vi "J1939 System Definition API_Example_Create Sysdef and Add J1939 CD.vi"(8 "error in (no error)":errorcluster) -> (0 "error out":errorcluster, 3 "Sysdef Path":path=path "C:/Users/Public/Documents/National Instruments/NI VeriStand 2011/Projects/DynamicallyCreatedProject/DynamicallyCreatedProject.nivssdf")   [LabVIEW 2013]
uses:
  J1939 System Definition API.lvlibp/APIs/System Definition API/Types/Add Item - Frame Cluster.ctl
  J1939 System Definition API.lvlibp/APIs/System Definition API/Types/Remove Frame Action.ctl
  J1939 System Definition API.lvlibp/Shared/Types/XNET Settings.ctl
  J1939 System Definition API.lvlibp/Shared/Types/Monitor Settings.ctl
  NationalInstruments.VeriStand.SystemDefinitionAPI
  J1939 System Definition API.lvlibp/APIs/System Definition API/SubVIs/Add Frames.vi
  J1939 System Definition API.lvlibp/APIs/System Definition API/SubVIs/Add Device.vi
  J1939 System Definition API.lvlibp/APIs/System Definition API/SubVIs/Add DTC.vi
  J1939 System Definition API.lvlibp
  J1939 System Definition API.lvlibp/APIs/System Definition API/J1939 System Definition API Support.lvlib
  J1939 System Definition API.lvlibp/Shared/J1939 Addon Shared.lvlib
panel:
  in  "Outgoing Frames":T1[](array[typedef])=[{"XNET Frame"="A1\nj1939", "Signals"=["EngBlowerBypassValvePos\nj1939", "EngGasSupplyPress\nj1939"]}, {"XNET Frame"="AAC1\nj1939", "Signals"=["Aftertreatment1AirPressCtrl\nj1939", "Aftertreatment1AirSystemRelay\nj1939", "Aftertreatment1PurgeAirActuator\nj1939", "Aftertreatment1PurgeAirPress\nj1939", "Aftertreatment1SupplyAirPress\nj1939", "Aftrtreatment1AirEnableActuator\nj1939", "Aftrtrtment1AirPressActuatorPos\nj1939", "Aftrtrtmnt1AtmzationAirActuator\nj1939"]}, {"XNET Frame"="AAC2\nj1939", "Signals"=["Aftertreatment2AirPressCtrl\nj1939", "Aftertreatment2AirSystemRelay\nj1939", "Aftertreatment2PurgeAirActuator\nj1939", "Aftertreatment2PurgeAirPress\nj1939", "Aftertreatment2SupplyAirPress\nj1939", "Aftrtreatment2AirEnableActuator\nj1939", "Aftrtrtment2AirPressActuatorPos\nj1939", "Aftrtrtmnt2AtmzationAirActuator\nj1939"]}, {"XNET Frame"="AAC3\nj1939", "Signals"=["Aftertreatment1SecondAirPress\nj1939", "Aftertreatment1SecondAirTemp\nj1939", "Aftrtratment1SecondAirDiffPress\nj1939", "Aftrtreatment1SecondAirMassFlow\nj1939"]}, {"XNET Frame"="AAC4\nj1939", "Signals"=["Aftertreatment2SecondAirPress\nj1939", "Aftertreatment2SecondAirTemp\nj1939", "Aftrtratment2SecondAirDiffPress\nj1939", "Aftrtreatment2SecondAirMassFlow\nj1939"]}, {"XNET Frame"="AAI\nj1939", "Signals"=["AuxLevel\nj1939", "AuxPress1\nj1939", "AuxPress2\nj1939", "AuxTemp1\nj1939", "AuxTemp2\nj1939"]}, {"XNET Frame"="AC\nj1939", "Signals"=["ArticulationAngle\nj1939"]}, {"XNET Frame"="ACC1\nj1939", "Signals"=["ACCDistanceAlertSignal\nj1939", "ACCSystemShutoffWarning\nj1939", "ACCTargetDetected\nj1939", "AdaptiveCruiseCtrlMode\nj1939", "AdaptiveCruiseCtrlSetSpeed\nj1939", "AdptveCruiseCtrlSetDistanceMode\nj1939", "DistanceToForwardVehicle\nj1939", "ACC1.RoadCurvature\nj1939", "SpeedOfForwardVehicle\nj1939"]}, {"XNET Frame"="ACC2\nj1939", "Signals"=["RqedACCDistanceMode\nj1939"]}, {"XNET Frame"="ACKM\nj1939", "Signals"=["AddressAccessDenied\nj1939", "AddressAcknowledged\nj1939", "AddressBusy\nj1939", "AddressNegativeAcknowledgement\nj1939", "ACKM.ControlByte\nj1939", "GroupFunctionValue\nj1939", "ACKM.ParameterGroupNumber\nj1939"]}, {"XNET Frame"="ACL\nj1939", "Signals"=["ACL.ArbitraryAddressCapable\nj1939", "ACL.ECUInstance\nj1939", "ACL.Function\nj1939", "ACL.FunctionInstance\nj1939", "ACL.IdentityNumber\nj1939", "ACL.IndustryGroup\nj1939", "ACL.ManufacturerCode\nj1939", "ACL.VehicleSystem\nj1939", "ACL.VehicleSystemInstance\nj1939"]}, {"XNET Frame"="AETC\nj1939", "Signals"=["AETCDataCollectionStandard\nj1939", "NumberOfAETCDataPoints\nj1939"]}, {"XNET Frame"="AF2\nj1939", "Signals"=["EngDsiredAbsIntakeManifoldPress\nj1939", "EngGasFuelCorrectionFactor\nj1939", "EngGsMssFlwSnsrFelingCorrection\nj1939", "EngTurboWastegateValvePos\nj1939"]}, {"XNET Frame"="AFC1\nj1939", "Signals"=["Aftertreatment1FuelPress\nj1939", "Aftertreatment1FuelPressCtrl\nj1939", "Aftertreatment1FuelRate\nj1939", "Aftertreatment1Ignt\nj1939", "Aftrtratment1FuelEnableActuator\nj1939", "Aftrtratment1RegenerationStatus\nj1939"]}, {"XNET Frame"="AFC2\nj1939", "Signals"=["Aftertreatment2FuelPress\nj1939", "Aftertreatment2FuelPressCtrl\nj1939", "Aftertreatment2FuelRate\nj1939", "Aftertreatment2Ignt\nj1939", "Aftrtratment2FuelEnableActuator\nj1939", "Aftrtratment2RegenerationStatus\nj1939"]}, {"XNET Frame"="AFSS\nj1939", "Signals"=["LeftHeadlampDynamicBendingLight\nj1939", "LeftHeadlampLightDistribution\nj1939", "RghtHeadlampDynamicBendingLight\nj1939", "RightHeadlampLightDistribution\nj1939"]}, {"XNET Frame"="AI\nj1939", "Signals"=["DriveAxleLiftAirPress\nj1939", "DriveAxleLocation\nj1939", "DriveAxleLubePress\nj1939", "DriveAxleTemp\nj1939", "SteerAxleLubePress\nj1939", "SteerAxleTemp\nj1939"]}, {"XNET Frame"="AIR1\nj1939", "Signals"=["AirCompressorStatus\nj1939", "AirSuspensionSupplyPress\nj1939", "AuxEquipmentSupplyPress\nj1939", "ParkingAnd_OrTrailerAirPress\nj1939", "PneumaticSupplyPress\nj1939", "ServiceBrakeAirPressCircuit1\nj1939", "ServiceBrakeAirPressCircuit2\nj1939"]}, {"XNET Frame"="AIR2\nj1939", "Signals"=["EngAirStartPress\nj1939"]}, {"XNET Frame"="AMB\nj1939", "Signals"=["AmbientAirTemp\nj1939", "BarometricPress\nj1939", "CabInteriorTemp\nj1939", "EngAirInletTemp\nj1939", "RoadSurfaceTemp\nj1939"]}, {"XNET Frame"="AMB2\nj1939", "Signals"=["SolarIntensityPercent\nj1939", "SolarSensorMax\nj1939"]}, {"XNET Frame"="AP\nj1939", "Signals"=["AuxAbsPressReading\nj1939", "AuxGagePressReading1\nj1939", "AuxVacuumPressReading\nj1939"]}, {"XNET Frame"="AS\nj1939", "Signals"=["Alt1Status\nj1939", "Alt2Status\nj1939", "Alt3Status\nj1939", "Alt4Status\nj1939", "AltSpeed\nj1939"]}, {"XNET Frame"="ASC1\nj1939", "Signals"=["AboveNominalLevelFrontAxle\nj1939", "AboveNominalLevelRearAxle\nj1939", "BelowNominalLevelFrontAxle\nj1939", "BelowNominalLevelRearAxle\nj1939", "DoorRelease\nj1939", "FrontAxleInBumperRange\nj1939", "KneelingInformation\nj1939", "LevelCtrlMode\nj1939", "ASC1.LiftAxle1Pos\nj1939", "ASC1.LiftAxle2Pos\nj1939", "LiftingCtrlModeFrontAxle\nj1939", "LiftingCtrlModeRearAxle\nj1939", "LoweringCtrlModeFrontAxle\nj1939", "LoweringCtrlModeRearAxle\nj1939", "NominalLevelFrontAxle\nj1939", "NominalLevelRearAxle\nj1939", "RearAxleInBumperRange\nj1939", "SecurityDevice\nj1939", "SspensionCtrlRefusalInformation\nj1939", "SuspensionRemoteCtrl1\nj1939", "SuspensionRemoteCtrl2\nj1939", "VehicleMotionInhibit\nj1939"]}, {"XNET Frame"="ASC2\nj1939", "Signals"=["AutomaticTractionHelp\nj1939", "DamperStiffnessRqFrontAxle\nj1939", "DamperStiffnessRqLift_TagAxle\nj1939", "DamperStiffnessRqRearAxle\nj1939", "KneelingCmdFrontAxle\nj1939", "KneelingCmdRearAxle\nj1939", "KneelingCtrlModeRq\nj1939", "KneelingRqLeftSide\nj1939", "KneelingRqRightSide\nj1939", "LevelCtrlModeRq\nj1939", "LiftAxle1PosCmd\nj1939", "LiftAxle2PosCmd\nj1939", "NominalLevelRqFrontAxle\nj1939", "NominalLevelRqRearAxle\nj1939", "ProhibitAirSuspensionCtrl\nj1939"]}, {"XNET Frame"="ASC3\nj1939", "Signals"=["RelativeLevelFrontAxleLeft\nj1939", "RelativeLevelFrontAxleRight\nj1939", "RelativeLevelRearAxleLeft\nj1939", "RelativeLevelRearAxleRight\nj1939"]}, {"XNET Frame"="ASC4\nj1939", "Signals"=["BellowPressFrontAxleLeft\nj1939", "BellowPressFrontAxleRight\nj1939", "BellowPressRearAxleLeft\nj1939", "BellowPressRearAxleRight\nj1939"]}, {"XNET Frame"="ASC5\nj1939", "Signals"=["DamperStiffnessFrontAxle\nj1939", "DamperStiffnessLift_TagAxle\nj1939", "DamperStiffnessRearAxle\nj1939", "ElctrncShckAbsrbrCtrlMdFrntAxle\nj1939", "ElctrncShckAbsrbrCtrlMdLft_TgAxl\nj1939", "ElctrncShckAbsrbrCtrlMdRearAxle\nj1939"]}, {"XNET Frame"="ASC6\nj1939", "Signals"=["LevelPresetFrontAxleLeft\nj1939", "LevelPresetFrontAxleRight\nj1939", "LevelPresetRearAxleLeft\nj1939", "LevelPresetRearAxleRight\nj1939"]}, {"XNET Frame"="AT\nj1939", "Signals"=["EngAltBearing1Temp\nj1939", "EngAltBearing2Temp\nj1939", "EngAltWinding1Temp\nj1939", "EngAltWinding2Temp\nj1939", "EngAltWinding3Temp\nj1939"]}, {"XNET Frame"="AT1I1\nj1939", "Signals"=["Aftertreatment1IntakeNOx\nj1939", "Aftertreatment1IntakeO2\nj1939", "Aftrtrtmnt1IntkGsSnsrHeaterCtrl\nj1939", "Aftrtrtmnt1IntkGsSnsrHtrPrlmnryF\nj1939", "Aftrtrtmnt1IntkGsSnsrPwrInRange\nj1939", "Aftrtrtmnt1IntkNOxReadingStable\nj1939", "Aftrtrtmnt1IntkNOxSnsrPrlmnryFMI\nj1939", "Aftrtrtmnt1IntkOxygnSnsrPrlmnryF\nj1939", "Aftrtrtmnt1IntkWdRngO2RdngStble\nj1939", "Aftrtrtmnt1IntkeGasSensorAtTemp\nj1939"]}, {"XNET Frame"="AT1I2\nj1939", "Signals"=["Aftertreatment1ExhaustGasTemp1\nj1939", "Aftrtrtmnt1ExhstGsTmp1PrlmnryFMI\nj1939", "Aftrtrtmnt1PrtcltTrpIntkGasTemp\nj1939", "Aftrtrtmnt1PrtcltTrpIntkGsTmpPrl\nj1939"]}, {"XNET Frame"="AT1O1\nj1939", "Signals"=["Aftertreatment1OutletNOx\nj1939", "Aftertreatment1OutletO2\nj1939", "Aftrtrtmnt1OtletGasSensorAtTemp\nj1939", "Aftrtrtmnt1OtltGsSnsrHeaterCtrl\nj1939", "Aftrtrtmnt1OtltGsSnsrHtrPrlmnryF\nj1939", "Aftrtrtmnt1OtltGsSnsrPwrInRange\nj1939", "Aftrtrtmnt1OtltNOxReadingStable\nj1939", "Aftrtrtmnt1OtltNOxSnsrPrlmnryFMI\nj1939", "Aftrtrtmnt1OtltOxygnSnsrPrlmnryF\nj1939", "Aftrtrtmnt1OtltWdRngO2RdngStble\nj1939"]}, {"XNET Frame"="AT1O2\nj1939", "Signals"=["Aftertreatment1ExhaustGasTemp3\nj1939", "Aftrtrtmnt1ExhstGsTmp3PrlmnryFMI\nj1939", "Aftrtrtmnt1PrtcltTrpOtltExhstGsT\nj1939", "Aftrtrtmnt1PrtcltTrpOtltGasTemp\nj1939"]}, {"XNET Frame"="AT2I1\nj1939", "Signals"=["Aftertreatment2IntakeNOx\nj1939", "Aftertreatment2IntakeO2\nj1939", "Aftrtrtmnt2IntkGsSnsrHeaterCtrl\nj1939", "Aftrtrtmnt2IntkGsSnsrHtrPrlmnryF\nj1939", "Aftrtrtmnt2IntkGsSnsrPwrInRange\nj1939", "Aftrtrtmnt2IntkNOxReadingStable\nj1939", "Aftrtrtmnt2IntkNOxSnsrPrlmnryFMI\nj1939", "Aftrtrtmnt2IntkOxygnSnsrPrlmnryF\nj1939", "Aftrtrtmnt2IntkWdRngO2RdngStble\nj1939", "Aftrtrtmnt2IntkeGasSensorAtTemp\nj1939"]}, {"XNET Frame"="AT2I2\nj1939", "Signals"=["Aftertreatment2ExhaustGasTemp1\nj1939", "Aftrtrtmnt2ExhstGsTmp1PrlmnryFMI\nj1939", "Aftrtrtmnt2PrtcltTrpIntkGasTemp\nj1939", "Aftrtrtmnt2PrtcltTrpIntkGsTmpPrl\nj1939"]}, {"XNET Frame"="AT2O1\nj1939", "Signals"=["Aftertreatment2OutletNOx\nj1939", "Aftertreatment2OutletO2\nj1939", "Aftrtrtmnt2OtletGasSensorAtTemp\nj1939", "Aftrtrtmnt2OtltGsSnsrHeaterCtrl\nj1939", "Aftrtrtmnt2OtltGsSnsrHtrPrlmnryF\nj1939", "Aftrtrtmnt2OtltGsSnsrPwrInRange\nj1939", "Aftrtrtmnt2OtltNOxReadingStable\nj1939", "Aftrtrtmnt2OtltNOxSnsrPrlmnryFMI\nj1939", "Aftrtrtmnt2OtltOxygnSnsrPrlmnryF\nj1939", "Aftrtrtmnt2OtltWdRngO2RdngStble\nj1939"]}, {"XNET Frame"="AT2O2\nj1939", "Signals"=["Aftertreatment2ExhaustGasTemp3\nj1939", "Aftrtrtmnt2ExhstGsTmp3PrlmnryFMI\nj1939", "Aftrtrtmnt2PrtcltTrpExhstGsTmpPr\nj1939", "Aftrtrtmnt2PrtcltTrpOtltGasTemp\nj1939"]}, {"XNET Frame"="ATGP1\nj1939", "Signals"=["ParticulateTrapIntakePress1\nj1939", "ParticulateTrapOutletPress1\nj1939"]}, {"XNET Frame"="ATGP2\nj1939", "Signals"=["ParticulateTrapIntakePress2\nj1939", "ParticulateTrapOutletPress2\nj1939"]}, {"XNET Frame"="ATM1\nj1939", "Signals"=["ExhaustGasTemp2\nj1939", "ExhaustGasTemp2PreliminaryFMI\nj1939", "ParticulateTrapDiffPress\nj1939", "PrtclateTrapIntermediateGasTemp\nj1939", "PrtcltTrpDltPressPreliminaryFMI\nj1939", "PrtcltTrpIntrmdtGsTmpPrlmnryFMI\nj1939"]}, {"XNET Frame"="ATM2\nj1939", "Signals"=["Aftertreatment2ExhaustGasTemp2\nj1939", "Aftrtrtmnt2ExhstGsTmp2PrlmnryFMI\nj1939", "Aftrtrtmnt2PrtcltTrpDltPrssPrlmn\nj1939", "Aftrtrtmnt2PrtcltTrpIntrmdtGsTmp\nj1939", "Aftrtrtmnt2PrtclteTrapDiffPress\nj1939"]}, {"XNET Frame"="ATR\nj1939", "Signals"=["AntitheftCmdStates\nj1939", "AntitheftDesiredExitModeStates\nj1939", "AntitheftPasswordRepresentation\nj1939", "AntthftEncryptonIndicatorStates\nj1939"]}, {"XNET Frame"="ATS\nj1939", "Signals"=["AntitheftComponentStatusStates\nj1939", "AntitheftModifyPwdStates\nj1939", "AntitheftPwdValidIndicator\nj1939", "AntitheftRandomNumber\nj1939", "AntthftEncryptnSdPrsntIndicator\nj1939"]}, {"XNET Frame"="ATS1\nj1939", "Signals"=["ParticulateTrap1AshLoadPercent\nj1939", "ParticulateTrap1SootLoadPercent\nj1939", "PrtcltTrp1TmSncLstActvRgnration\nj1939"]}, {"XNET Frame"="ATS2\nj1939", "Signals"=["ParticulateTrap2AshLoadPercent\nj1939", "ParticulateTrap2SootLoadPercent\nj1939", "PrtcltTrp2TmSncLstActvRgnration\nj1939"]}, {"XNET Frame"="AUXIO1\nj1939", "Signals"=["AuxI_OChannel1\nj1939", "AuxI_OChannel2\nj1939"]}, {"XNET Frame"="AUXIO2\nj1939", "Signals"=["AuxI_O17\nj1939", "AuxI_O18\nj1939", "AuxI_O19\nj1939", "AuxI_O20\nj1939", "AuxI_O21\nj1939", "AuxI_O22\nj1939", "AuxI_O23\nj1939", "AuxI_O24\nj1939", "AuxI_O25\nj1939", "AuxI_O26\nj1939", "AuxI_O27\nj1939", "AuxI_O28\nj1939", "AuxI_O29\nj1939", "AuxI_O30\nj1939", "AuxI_O31\nj1939", "AuxI_O32\nj1939", "AuxI_O33\nj1939", "AuxI_O34\nj1939", "AuxI_O35\nj1939", "AuxI_O36\nj1939", "AuxI_O37\nj1939", "AuxI_O38\nj1939", "AuxI_O39\nj1939", "AuxI_O40\nj1939", "AuxI_O41\nj1939", "AuxI_O42\nj1939", "AuxI_O43\nj1939", "AuxI_O44\nj1939", "AuxI_O45\nj1939", "AuxI_O46\nj1939", "AuxI_O47\nj1939", "AuxI_O48\nj1939"]}, {"XNET Frame"="AUXIO3\nj1939", "Signals"=["AuxI_O49\nj1939", "AuxI_O50\nj1939", "AuxI_O51\nj1939", "AuxI_O52\nj1939", "AuxI_O53\nj1939", "AuxI_O54\nj1939", "AuxI_O55\nj1939", "AuxI_O56\nj1939", "AuxI_O57\nj1939", "AuxI_O58\nj1939", "AuxI_O59\nj1939", "AuxI_O60\nj1939", "AuxI_O61\nj1939", "AuxI_O62\nj1939", "AuxI_O63\nj1939", "AuxI_O64\nj1939", "AuxI_O65\nj1939", "AuxI_O66\nj1939", "AuxI_O67\nj1939", "AuxI_O68\nj1939", "AuxI_O69\nj1939", "AuxI_O70\nj1939", "AuxI_O71\nj1939", "AuxI_O72\nj1939", "AuxI_O73\nj1939", "AuxI_O74\nj1939", "AuxI_O75\nj1939", "AuxI_O76\nj1939", "AuxI_O77\nj1939", "AuxI_O78\nj1939", "AuxI_O79\nj1939", "AuxI_O80\nj1939"]}, {"XNET Frame"="AUXIO4\nj1939", "Signals"=["AuxI_O100\nj1939", "AuxI_O101\nj1939", "AuxI_O102\nj1939", "AuxI_O103\nj1939", "AuxI_O104\nj1939", "AuxI_O105\nj1939", "AuxI_O106\nj1939", "AuxI_O107\nj1939", "AuxI_O108\nj1939", "AuxI_O109\nj1939", "AuxI_O110\nj1939", "AuxI_O111\nj1939", "AuxI_O112\nj1939", "AuxI_O81\nj1939", "AuxI_O82\nj1939", "AuxI_O83\nj1939", "AuxI_O84\nj1939", "AuxI_O85\nj1939", "AuxI_O86\nj1939", "AuxI_O87\nj1939", "AuxI_O88\nj1939", "AuxI_O89\nj1939", "AuxI_O90\nj1939", "AuxI_O91\nj1939", "AuxI_O92\nj1939", "AuxI_O93\nj1939", "AuxI_O94\nj1939", "AuxI_O95\nj1939", "AuxI_O96\nj1939", "AuxI_O97\nj1939", "AuxI_O98\nj1939", "AuxI_O99\nj1939"]}, {"XNET Frame"="AWPP\nj1939", "Signals"=["AuxPumpPress\nj1939"]}, {"XNET Frame"="B\nj1939", "Signals"=["BrakeAppPress\nj1939", "BrakePrimaryPress\nj1939", "BrakeSecondPress\nj1939", "ParkBrakeReleaseInhibitStatus\nj1939", "ParkingBrakeActuator\nj1939", "ParkingBrakeRedWarningSignal\nj1939"]}, {"XNET Frame"="BAAC\nj1939", "Signals"=["Bs1AvrgeLineNeutralACRMSVoltage\nj1939", "Bus1AverageACFrequency\nj1939", "Bus1AverageLineLineACRMSVoltage\nj1939"]}, {"XNET Frame"="BGSC\nj1939", "Signals"=["Bus1_GeneratorACPhaseDifference\nj1939", "Bus1_GeneratorDeadBus\nj1939", "Bus1_GeneratorFrequencyMatch\nj1939", "Bus1_GeneratorInSync\nj1939", "Bus1_GeneratorPhaseMatch\nj1939", "Bus1_GeneratorVoltageMatch\nj1939"]}, {"XNET Frame"="BI\nj1939", "Signals"=["BladeRotationAngle\nj1939", "BladeRotationAngleFigureOfMerit\nj1939", "RelBladeHeightFigureOfMerit\nj1939", "RelBladeMeasurementLatency\nj1939", "RelativeBladeHeight\nj1939"]}, {"XNET Frame"="BJM1\nj1939", "Signals"=["Joystick1Button10PressedStatus\nj1939", "Joystick1Button11PressedStatus\nj1939", "Joystick1Button12PressedStatus\nj1939", "Joystick1Button1PressedStatus\nj1939", "Joystick1Button2PressedStatus\nj1939", "Joystick1Button3PressedStatus\nj1939", "Joystick1Button4PressedStatus\nj1939", "Joystick1Button5PressedStatus\nj1939", "Joystick1Button6PressedStatus\nj1939", "Joystick1Button7PressedStatus\nj1939", "Joystick1Button8PressedStatus\nj1939", "Joystick1Button9PressedStatus\nj1939", "Joystick1XAxisDetentPosStatus\nj1939", "Joystick1XAxisNeutralPosStatus\nj1939", "Joystick1XAxisPos\nj1939", "Joystick1YAxisDetentPosStatus\nj1939", "Joystick1YAxisNeutralPosStatus\nj1939", "Joystick1YAxisPos\nj1939", "Jystck1XAxsLvrLftNgtvePosStatus\nj1939", "Jystck1XAxsLvrRghtPstvPosStatus\nj1939", "Jystck1YAxsLvrBckNgtvePosStatus\nj1939", "Jystck1YAxsLvrFrwrdPstvPsStatus\nj1939"]}, {"XNET Frame"="BJM2\nj1939", "Signals"=["Joystick2Button10PressedStatus\nj1939", "Joystick2Button11PressedStatus\nj1939", "Joystick2Button12PressedStatus\nj1939", "Joystick2Button1PressedStatus\nj1939", "Joystick2Button2PressedStatus\nj1939", "Joystick2Button3PressedStatus\nj1939", "Joystick2Button4PressedStatus\nj1939", "Joystick2Button5PressedStatus\nj1939", "Joystick2Button6PressedStatus\nj1939", "Joystick2Button7PressedStatus\nj1939", "Joystick2Button8PressedStatus\nj1939", "Joystick2Button9PressedStatus\nj1939", "Joystick2XAxisDetentPosStatus\nj1939", "Joystick2XAxisNeutralPosStatus\nj1939", "Joystick2XAxisPos\nj1939", "Joystick2YAxisDetentPosStatus\nj1939", "Joystick2YAxisNeutralPosStatus\nj1939", "Joystick2YAxisPos\nj1939", "Jystck2XAxsLvrLftNgtvePosStatus\nj1939", "Jystck2XAxsLvrRghtPstvPosStatus\nj1939", "Jystck2YAxsLvrBckNgtvePosStatus\nj1939", "Jystck2YAxsLvrFrwrdPstvPsStatus\nj1939"]}, {"XNET Frame"="BJM3\nj1939", "Signals"=["Joystick3Button10PressedStatus\nj1939", "Joystick3Button11PressedStatus\nj1939", "Joystick3Button12PressedStatus\nj1939", "Joystick3Button1PressedStatus\nj1939", "Joystick3Button2PressedStatus\nj1939", "Joystick3Button3PressedStatus\nj1939", "Joystick3Button4PressedStatus\nj1939", "Joystick3Button5PressedStatus\nj1939", "Joystick3Button6PressedStatus\nj1939", "Joystick3Button7PressedStatus\nj1939", "Joystick3Button8PressedStatus\nj1939", "Joystick3Button9PressedStatus\nj1939", "Joystick3XAxisDetentPosStatus\nj1939", "Joystick3XAxisNeutralPosStatus\nj1939", "Joystick3XAxisPos\nj1939", "Joystick3YAxisDetentPosStatus\nj1939", "Joystick3YAxisNeutralPosStatus\nj1939", "Joystick3YAxisPos\nj1939", "Jystck3XAxsLvrLftNgtvePosStatus\nj1939", "Jystck3XAxsLvrRghtPstvPosStatus\nj1939", "Jystck3YAxsLvrBckNgtvePosStatus\nj1939", "Jystck3YAxsLvrFrwrdPstvPsStatus\nj1939"]}, {"XNET Frame"="BM\nj1939", "Signals"=["BatteryMainSwitchHoldState\nj1939"]}, {"XNET Frame"="BPAAC\nj1939", "Signals"=["Bs1PhseALineNeutralACRMSVoltage\nj1939", "Bus1PhaseAACFrequency\nj1939", "Bus1PhaseABLineLineACRMSVoltage\nj1939"]}, {"XNET Frame"="BPBAC\nj1939", "Signals"=["Bs1PhseBLineNeutralACRMSVoltage\nj1939", "Bus1PhaseBACFrequency\nj1939", "Bus1PhaseBCLineLineACRMSVoltage\nj1939"]}, {"XNET Frame"="BPCAC\nj1939", "Signals"=["Bs1PhseCLineNeutralACRMSVoltage\nj1939", "Bus1PhaseCACFrequency\nj1939", "Bus1PhaseCALineLineACRMSVoltage\nj1939"]}, {"XNET Frame"="BSA\nj1939", "Signals"=["TractorBrakeStrokeAxle1Left\nj1939", "TractorBrakeStrokeAxle1Right\nj1939", "TractorBrakeStrokeAxle2Left\nj1939", "TractorBrakeStrokeAxle2Right\nj1939", "TractorBrakeStrokeAxle3Left\nj1939", "TractorBrakeStrokeAxle3Right\nj1939", "TractorBrakeStrokeAxle4Left\nj1939", "TractorBrakeStrokeAxle4Right\nj1939", "TractorBrakeStrokeAxle5Left\nj1939", "TractorBrakeStrokeAxle5Right\nj1939", "TrailerBrakeStrokeAxle1Left\nj1939", "TrailerBrakeStrokeAxle1Right\nj1939", "TrailerBrakeStrokeAxle2Left\nj1939", "TrailerBrakeStrokeAxle2Right\nj1939", "TrailerBrakeStrokeAxle3Left\nj1939", "TrailerBrakeStrokeAxle3Right\nj1939", "TrailerBrakeStrokeAxle4Left\nj1939", "TrailerBrakeStrokeAxle4Right\nj1939", "TrailerBrakeStrokeAxle5Left\nj1939", "TrailerBrakeStrokeAxle5Right\nj1939"]}, {"XNET Frame"="BT1\nj1939", "Signals"=["Battery1Temp\nj1939", "Battery2Temp\nj1939"]}, {"XNET Frame"="BUSC\nj1939", "Signals"=["Bus1_UtilityACPhaseDifference\nj1939", "Bus1_UtilityDeadBus\nj1939", "Bus1_UtilityFrequencyMatch\nj1939", "Bus1_UtilityInSync\nj1939", "Bus1_UtilityPhaseMatch\nj1939", "Bus1_UtilityVoltageMatch\nj1939"]}, {"XNET Frame"="CACI\nj1939", "Signals"=["CbA_CRfrgrntCmprssorOutletPress\nj1939"]}, {"XNET Frame"="CCC\nj1939", "Signals"=["AuxHeaterMaxOutputPower\nj1939"]}, {"XNET Frame"="CCS\nj1939", "Signals"=["EngCyl10CombustionStatus\nj1939", "EngCyl11CombustionStatus\nj1939", "EngCyl12CombustionStatus\nj1939", "EngCyl13CombustionStatus\nj1939", "EngCyl14CombustionStatus\nj1939", "EngCyl15CombustionStatus\nj1939", "EngCyl16CombustionStatus\nj1939", "EngCyl17CombustionStatus\nj1939", "EngCyl18CombustionStatus\nj1939", "EngCyl19CombustionStatus\nj1939", "EngCyl1CombustionStatus\nj1939", "EngCyl20CombustionStatus\nj1939", "EngCyl21CombustionStatus\nj1939", "EngCyl22CombustionStatus\nj1939", "EngCyl23CombustionStatus\nj1939", "EngCyl24CombustionStatus\nj1939", "EngCyl2CombustionStatus\nj1939", "EngCyl3CombustionStatus\nj1939", "EngCyl4CombustionStatus\nj1939", "EngCyl5CombustionStatus\nj1939", "EngCyl6CombustionStatus\nj1939", "EngCyl7CombustionStatus\nj1939", "EngCyl8CombustionStatus\nj1939", "EngCyl9CombustionStatus\nj1939"]}, {"XNET Frame"="CCSS\nj1939", "Signals"=["CruiseCtrlHighSetLimitSpeed\nj1939", "CruiseCtrlLowSetLimitSpeed\nj1939", "CCSS.MaxVehicleSpeedLimit\nj1939"]}, {"XNET Frame"="CCVS\nj1939", "Signals"=["BrakeSwitch\nj1939", "ClutchSwitch\nj1939", "CruiseCtrlAccelerateSwitch\nj1939", "CruiseCtrlActive\nj1939", "CruiseCtrlCoastSwitch\nj1939", "CruiseCtrlEnableSwitch\nj1939", "CruiseCtrlPauseSwitch\nj1939", "CruiseCtrlResumeSwitch\nj1939", "CruiseCtrlSetSpeed\nj1939", "CruiseCtrlSetSwitch\nj1939", "CruiseCtrlStates\nj1939", "EngIdleDecrementSwitch\nj1939", "EngIdleIncrementSwitch\nj1939", "EngShutdownOverrideSwitch\nj1939", "EngTestModeSwitch\nj1939", "PTOState\nj1939", "ParkBrakeReleaseInhibitRq\nj1939", "ParkingBrakeSwitch\nj1939", "TwoSpeedAxleSwitch\nj1939", "CCVS.WheelBasedVehicleSpeed\nj1939"]}, {"XNET Frame"="CL\nj1939", "Signals"=["IlluminationBrightnessPercent\nj1939"]}, {"XNET Frame"="CM1\nj1939", "Signals"=["AtmaticGearShiftingEnableSwitch\nj1939", "AuxHeaterCoolantPumpRq\nj1939", "AuxHeaterModeRq\nj1939", "BatteryMainSwitchHoldRq\nj1939", "CabInteriorTempCmd\nj1939", "EngAutomaticStartEnableSwitch\nj1939", "OperatorSeatDirectionSwitch\nj1939", "RqCabZoneHeating\nj1939", "RqEngZoneHeating\nj1939", "RqedPercentFanSpeed\nj1939", "SeatBeltSwitch\nj1939", "SelectedMaxVehicleSpeedLimit\nj1939", "VhclLmtngSpdGvernorEnableSwitch\nj1939", "VhclLmtngSpdGvrnrDcrementSwitch\nj1939", "VhclLmtngSpdGvrnrIncrmentSwitch\nj1939"]}, {"XNET Frame"="CM3\nj1939", "Signals"=["FfthWhlRlaseCtrlSecurityLockout\nj1939", "FifthWheelReleaseCtrl\nj1939", "TransOilLevelRq\nj1939", "TransferCaseSelectorSwitch\nj1939"]}, {"XNET Frame"="CMI\nj1939", "Signals"=["TotalCountOfConfigChangesMade\nj1939"]}, {"XNET Frame"="CRI1\nj1939", "Signals"=["CatalystReagentConcentration\nj1939", "CatalystReagentConductivity\nj1939", "CatalystReagentTemp2\nj1939", "CatalystReagentType\nj1939", "CtlystRagentTemp2PreliminaryFMI\nj1939", "CtlystRgntPrprtesPreliminaryFMI\nj1939"]}, {"XNET Frame"="CSA\nj1939", "Signals"=["EngStartEnableDevice1\nj1939", "EngStartEnableDevice1Config\nj1939", "EngStartEnableDevice2\nj1939", "EngStartEnableDevice2Config\nj1939"]}, {"XNET Frame"="CT1\nj1939", "Signals"=["EngCyl1CombustionTime\nj1939", "EngCyl2CombustionTime\nj1939", "EngCyl3CombustionTime\nj1939", "EngCyl4CombustionTime\nj1939"]}, {"XNET Frame"="CT2\nj1939", "Signals"=["EngCyl5CombustionTime\nj1939", "EngCyl6CombustionTime\nj1939", "EngCyl7CombustionTime\nj1939", "EngCyl8CombustionTime\nj1939"]}, {"XNET Frame"="CT3\nj1939", "Signals"=["EngCyl10CombustionTime\nj1939", "EngCyl11CombustionTime\nj1939", "EngCyl12CombustionTime\nj1939", "EngCyl9CombustionTime\nj1939"]}, {"XNET Frame"="CT4\nj1939", "Signals"=["EngCyl13CombustionTime\nj1939", "EngCyl14CombustionTime\nj1939", "EngCyl15CombustionTime\nj1939", "EngCyl16CombustionTime\nj1939"]}, {"XNET Frame"="CT5\nj1939", "Signals"=["EngCyl17CombustionTime\nj1939", "EngCyl18CombustionTime\nj1939", "EngCyl19CombustionTime\nj1939", "EngCyl20CombustionTime\nj1939"]}, {"XNET Frame"="CT6\nj1939", "Signals"=["EngAverageCombustionTime\nj1939", "EngDesiredCombustionTime\nj1939"]}, {"XNET Frame"="CTL\nj1939", "Signals"=["EngSpeedLimitRqMaxContinuous\nj1939", "EngSpeedLimitRqMinContinuous\nj1939", "EngTorqueLimitRqMaxContinuous\nj1939", "EngTorqueLimitRqMinContinuous\nj1939", "MnCntinuousRetarderSpeedLimitRq\nj1939", "MnCntnuousRetarderTorqueLimitRq\nj1939", "MxCntinuousRetarderSpeedLimitRq\nj1939", "MxCntnuousRetarderTorqueLimitRq\nj1939"]}, {"XNET Frame"="CVW\nj1939", "Signals"=["GrossCombinationVehicleWeight\nj1939", "PoweredVehicleWeight\nj1939"]}, {"XNET Frame"="DC1\nj1939", "Signals"=["PosOfDoors\nj1939", "Ramp_WheelChairLiftPos\nj1939", "Status2OfDoors\nj1939"]}, {"XNET Frame"="DC2\nj1939", "Signals"=["EnableStatusOfDoor1\nj1939", "EnableStatusOfDoor10\nj1939", "EnableStatusOfDoor2\nj1939", "EnableStatusOfDoor3\nj1939", "EnableStatusOfDoor4\nj1939", "EnableStatusOfDoor5\nj1939", "EnableStatusOfDoor6\nj1939", "EnableStatusOfDoor7\nj1939", "EnableStatusOfDoor8\nj1939", "EnableStatusOfDoor9\nj1939", "LockStatusOfDoor1\nj1939", "LockStatusOfDoor10\nj1939", "LockStatusOfDoor2\nj1939", "LockStatusOfDoor3\nj1939", "LockStatusOfDoor4\nj1939", "LockStatusOfDoor5\nj1939", "LockStatusOfDoor6\nj1939", "LockStatusOfDoor7\nj1939", "LockStatusOfDoor8\nj1939", "LockStatusOfDoor9\nj1939", "OpenStatusOfDoor1\nj1939", "OpenStatusOfDoor10\nj1939", "OpenStatusOfDoor2\nj1939", "OpenStatusOfDoor3\nj1939", "OpenStatusOfDoor4\nj1939", "OpenStatusOfDoor5\nj1939", "OpenStatusOfDoor6\nj1939", "OpenStatusOfDoor7\nj1939", "OpenStatusOfDoor8\nj1939", "OpenStatusOfDoor9\nj1939"]}, {"XNET Frame"="DD\nj1939", "Signals"=["CargoAmbientTemp\nj1939", "EngFuelFilterDiffPress\nj1939", "EngOilFilterDiffPress\nj1939", "FuelLevel\nj1939", "WasherFluidLevel\nj1939"]}, {"XNET Frame"="DISP1\nj1939", "Signals"=["TextDisplayIndex\nj1939", "TextDisplayInstructions\nj1939"]}, {"XNET Frame"="DM10\nj1939", "Signals"=["TestIdentifierSupported\nj1939"]}, {"XNET Frame"="DM13\nj1939", "Signals"=["CurrentDataLink\nj1939", "HoldSignal\nj1939", "ISO9141\nj1939", "J1939Network1\nj1939", "J1939Network2\nj1939", "J1939Network3\nj1939", "ManufacturerSpecificPort\nj1939", "SAE_J1587\nj1939", "SAE_J1850\nj1939", "SAE_J1922\nj1939", "SuspendDuration\nj1939", "SuspendSignal\nj1939"]}, {"XNET Frame"="DM14\nj1939", "Signals"=["Command\nj1939", "KeyOrUserLevel\nj1939", "NumberRequested\nj1939", "NumberRequestedHigh\nj1939", "Pointer\nj1939", "PointerExtension\nj1939", "PointerType\nj1939"]}, {"XNET Frame"="DM15\nj1939", "Signals"=["EDCP_Extension\nj1939", "ErrorIndicator\nj1939", "NumberAllowed\nj1939", "NumberAllowedHigh\nj1939", "Seed\nj1939", "Status\nj1939"]}, {"XNET Frame"="DM16\nj1939", "Signals"=["NumberOfOccurance\nj1939"]}, {"XNET Frame"="DM18\nj1939", "Signals"=["SecurityEntityLength\nj1939", "SecurityEntityLengthHigh\nj1939", "SecurityEntityType\nj1939"]}, {"XNET Frame"="DM21\nj1939", "Signals"=["DistanceSinceDTCsCleared\nj1939", "DistanceWhileMILisActivated\nj1939", "MinutesRunByEngineMILActivated\nj1939", "TimeSinceDTCsCleared\nj1939"]}, {"XNET Frame"="DM22\nj1939", "Signals"=["CtrlByteIndicIndividualDTCClear\nj1939", "DM22.FailureModeIdentifier1\nj1939", "IndividualDTCClearControlByte\nj1939", "DM22.SPN1\nj1939", "DM22.SPN1High\nj1939"]}, {"XNET Frame"="DM26\nj1939", "Signals"=["ACSystemRefrigerantMonComplete\nj1939", "ACSystemRefrigerantMonEnabled\nj1939", "CatalystMonComplete\nj1939", "CatalystMonEnabled\nj1939", "ColdStartAidSystemMonComplete\nj1939", "ColdStartAidSystemMonEnabled\nj1939", "ComprehensiveCompMonEnabled\nj1939", "ComprehensiveComptMonComplete\nj1939", "EGRSystemMonitoringComplete\nj1939", "EGRSystemMonitoringEnabled\nj1939", "EvaporativeSystemMonComplete\nj1939", "EvaporativeSystemMonEnabled\nj1939", "FuelSystemMonitoringComplete\nj1939", "FuelSystemMonitoringEnabled\nj1939", "HeatedCatalystMonComplete\nj1939", "HeatedCatalystMonEnabled\nj1939", "MisfireMonitoringComplete\nj1939", "MisfireMonitoringEnabled\nj1939", "NumOfWarmUpsSinceDTCsCleared\nj1939", "OxygenSensorHeaterMonComplete\nj1939", "OxygenSensorHeaterMonEnabled\nj1939", "OxygenSensorMonComplete\nj1939", "OxygenSensorMonEnabled\nj1939", "SecondAirSystemMonComplete\nj1939", "SecondAirSystemMonEnabled\nj1939", "TimeSinceEngineStart\nj1939"]}, {"XNET Frame"="DM29\nj1939", "Signals"=["AllPendingDTCs\nj1939", "MILOnDTCs\nj1939", "PendingDTCs\nj1939", "PermanentDTCs\nj1939", "PreviouslyMILOnDTCs\nj1939"]}, {"XNET Frame"="DM5\nj1939", "Signals"=["ACSystemRefrigerantMonStatus\nj1939", "ACSystemRefrigerantMonSupp\nj1939", "ActiveTroubleCodes\nj1939", "CatalystMonStatus\nj1939", "CatalystMonSupp\nj1939", "ColdStartAidSystemMonStatus\nj1939", "ColdStartAidSystemMonSupp\nj1939", "ComprehensiveCompMonStatus\nj1939", "ComprehensiveComponentMonSupp\nj1939", "EGRSystemMonitoringStatus\nj1939", "EGRSystemMonitoringSupp\nj1939", "EvaporativeSystemMonStatus\nj1939", "EvaporativeSystemMonSupp\nj1939", "FuelSystemMonitoringStatus\nj1939", "FuelSystemMonitoringSupport\nj1939", "HeatedCatalystMonStatus\nj1939", "HeatedCatalystMonSupp\nj1939", "MisfireMonitoringStatus\nj1939", "MisfireMonitoringSupport\nj1939", "OBDCompliance\nj1939", "OxygenSensorHeaterMonStatus\nj1939", "OxygenSensorHeaterMonSupp\nj1939", "OxygenSensorMonStatus\nj1939", "OxygenSensorMonSupp\nj1939", "PreviouslyActiveTroubleCodes\nj1939", "SecondAirSystemMonStatus\nj1939", "SecondAirSystemMonSupp\nj1939"]}, {"XNET Frame"="DM7\nj1939", "Signals"=["DM7.TestIdentifier\nj1939"]}, {"XNET Frame"="DM8\nj1939", "Signals"=["DM8.TestIdentifier\nj1939", "TestLimitMaximum\nj1939", "TestLimitMinimum\nj1939", "TestType\nj1939", "TestValue\nj1939"]}, {"XNET Frame"="DRC\nj1939", "Signals"=["EnableStatusOfRamp1\nj1939", "EnableStatusOfRamp2\nj1939", "EnableStatusOfRamp3\nj1939", "MovementStatusOfRamp1\nj1939", "MovementStatusOfRamp2\nj1939", "MovementStatusOfRamp3\nj1939", "RetractStatusOfRamp1\nj1939", "RetractStatusOfRamp2\nj1939", "RetractStatusOfRamp3\nj1939"]}, {"XNET Frame"="EAC\nj1939", "Signals"=["EngAuxCoolantPress\nj1939", "EngAuxCoolantTemp\nj1939", "SeaWaterPumpOutletPress\nj1939"]}, {"XNET Frame"="EAC1\nj1939", "Signals"=["DiffLockStateCentral\nj1939", "DiffLockStateCentralFront\nj1939", "DiffLockStateCentralRear\nj1939", "DiffLockStateFrontAxle1\nj1939", "DiffLockStateFrontAxle2\nj1939", "DiffLockStateRearAxle1\nj1939", "DiffLockStateRearAxle2\nj1939", "FrontAxleGroupEngagementStatus\nj1939", "Location\nj1939", "RearAxleGroupEngagementStatus\nj1939"]}, {"XNET Frame"="EBC1\nj1939", "Signals"=["ABSFullyOperational\nj1939", "ABSOffroadSwitch\nj1939", "ABS_EBSAmberWarningSignal\nj1939", "ASRBrakeCtrlActive\nj1939", "ASREngCtrlActive\nj1939", "ASRHillHolderSwitch\nj1939", "ASROffroadSwitch\nj1939", "ATC_ASRInformationSignal\nj1939", "AccelInterlockSwitch\nj1939", "AntiLockBrakingActive\nj1939", "BrakePedalPos\nj1939", "EBSBrakeSwitch\nj1939", "EBSRedWarningSignal\nj1939", "EngAuxEngShutdownSwitch\nj1939", "EngDerateSwitch\nj1939", "EngRetarderSelection\nj1939", "HaltBrakeSwitch\nj1939", "RemoteAccelEnableSwitch\nj1939", "SrcAddrssOfCtrllngDvcFrBrkCntrl\nj1939", "TractionCtrlOverrideSwitch\nj1939", "TrailerABSStatus\nj1939", "TrctrMntdTrilerABSWarningSignal\nj1939"]}, {"XNET Frame"="EBC2\nj1939", "Signals"=["FrontAxleSpeed\nj1939", "RelativeSpeedFrontAxleLeftWheel\nj1939", "RelativeSpeedRearAxle1LeftWheel\nj1939", "RelativeSpeedRearAxle2LeftWheel\nj1939", "RlativeSpeedFrontAxleRightWheel\nj1939", "RlativeSpeedRearAxle1RightWheel\nj1939", "RlativeSpeedRearAxle2RightWheel\nj1939"]}, {"XNET Frame"="EBC3\nj1939", "Signals"=["BrkAppPrssHghRngFrntAxlLftWheel\nj1939", "BrkAppPrssHghRngFrntAxlRghtWhel\nj1939", "BrkAppPrssHghRngRrAxl1LeftWheel\nj1939", "BrkAppPrssHghRngRrAxl1RghtWheel\nj1939", "BrkAppPrssHghRngRrAxl2LeftWheel\nj1939", "BrkAppPrssHghRngRrAxl2RghtWheel\nj1939", "BrkAppPrssHghRngRrAxl3LeftWheel\nj1939", "BrkAppPrssHghRngRrAxl3RghtWheel\nj1939"]}, {"XNET Frame"="EBC4\nj1939", "Signals"=["BrkLnngRmningFrontAxleLeftWheel\nj1939", "BrkLnngRmningRearAxle1LeftWheel\nj1939", "BrkLnngRmningRearAxle2LeftWheel\nj1939", "BrkLnngRmningRearAxle3LeftWheel\nj1939", "BrkLnngRmnngFrontAxleRightWheel\nj1939", "BrkLnngRmnngRearAxle1RightWheel\nj1939", "BrkLnngRmnngRearAxle2RightWheel\nj1939", "BrkLnngRmnngRearAxle3RightWheel\nj1939"]}, {"XNET Frame"="EBC5\nj1939", "Signals"=["BrakeTempWarning\nj1939", "FoundationBrakeUse\nj1939", "HaltBrakeMode\nj1939", "HillHolderMode\nj1939", "XBRAccelerationLimit\nj1939", "XBRActiveCtrlMode\nj1939", "XBRSystemState\nj1939"]}, {"XNET Frame"="EBS11\nj1939", "Signals"=["ASRBreakControlActive\nj1939", "ASREngineControlActive\nj1939", "BrakeLightSwitch\nj1939", "ParkBrakeDemandValue\nj1939", "RetarderDemandValue\nj1939", "ServiceBrakeDemandValue\nj1939", "EBS11.VehicleABSActive\nj1939", "EBS11.VehicleRetarderCtrlActive\nj1939", "EBS11.VehicleType\nj1939"]}, {"XNET Frame"="EBS12\nj1939", "Signals"=["ABSOffroadRequest\nj1939", "PneumaticControlLine\nj1939", "EBS12.RoadCurvature\nj1939", "TwoElCircuitsBrakeDemand\nj1939", "EBS12.VehicleRetarderCtrlActive\nj1939"]}, {"XNET Frame"="EBS21\nj1939", "Signals"=["ActualRetarderPercTorque\nj1939", "EBS21.AutomTowedVehBreakActive\nj1939", "EBS21.SupplyLineBrakingRequest\nj1939", "VDCActive\nj1939", "EBS21.VehicleABSActive\nj1939", "EBS21.VehicleRetarderCtrlActive\nj1939", "EBS21.VehicleServiceBrakeActive\nj1939", "WheelSpeedDiffMainAxle\nj1939", "Wheel_BasedVehicleSpeed\nj1939"]}, {"XNET Frame"="EBS22\nj1939", "Signals"=["AmberWarningSignalReq\nj1939", "EBS22.AutomTowedVehBreakActive\nj1939", "AxleLoadSum\nj1939", "ElecSupplyOfNonBrakingSys\nj1939", "ElectrLoadPropFunc\nj1939", "LoadingRampApproachAssist\nj1939", "RedWarningSignalRequest\nj1939", "EBS22.ReferenceRetarderTorque\nj1939", "SpringBrakeEngaged\nj1939", "SpringBrakeInstalled\nj1939", "EBS22.SupplyLineBrakingRequest\nj1939", "EBS22.VehicleABSActive\nj1939", "VehicleElectrSupplySuff\nj1939", "EBS22.VehicleRetarderCtrlActive\nj1939", "EBS22.VehicleServiceBrakeActive\nj1939", "EBS22.VehicleType\nj1939"]}, {"XNET Frame"="EBS23\nj1939", "Signals"=["BrakeLining\nj1939", "BrakeLiningSufficient\nj1939", "BrakeTemperature\nj1939", "BrakeTemperatureStatus\nj1939", "PneumaticSupplyPressure\nj1939", "TyrePressure\nj1939", "TyrePressureSufficient\nj1939", "TyreWheelIdentLining1\nj1939", "TyreWheelIdentLining2\nj1939", "TyreWheelIdentPressure1\nj1939", "TyreWheelIdentPressure2\nj1939", "TyreWheelIdentTemp1\nj1939", "TyreWheelIdentTemp2\nj1939", "VehiclePneumSupplySuff\nj1939"]}, {"XNET Frame"="EC2\nj1939", "Signals"=["MaxCrankAttemptsPerStartAttempt\nj1939"]}, {"XNET Frame"="ECT1\nj1939", "Signals"=["EngHghLmtThrshhldFrMnCntnsEngRPM\nj1939", "EngHghLmtThrshhldFrMnCntnsTrqFrm\nj1939", "EngLwLmtThrshhldFrMaxRPMFromEng\nj1939", "EngLwLmtThrshldFrMxTrqueFromEng\nj1939", "EngMaxContinuousRPM\nj1939", "EngMaxContinuousTorque\nj1939", "EngMinContinuousRPM\nj1939", "EngMinContinuousTorque\nj1939"]}, {"XNET Frame"="EEC1\nj1939", "Signals"=["ActualEngPercentTorque\nj1939", "DriversDemandEngPercentTorque\nj1939", "EngDemandPercentTorque\nj1939", "EEC1.EngSpeed\nj1939", "EngStarterMode\nj1939", "EEC1.EngTorqueMode\nj1939", "SrcAddrssOfCtrllngDvcForEngCtrl\nj1939"]}, {"XNET Frame"="EEC2\nj1939", "Signals"=["AccelPedal1LowIdleSwitch\nj1939", "AccelPedal2LowIdleSwitch\nj1939", "AccelPedalKickdownSwitch\nj1939", "AccelPedalPos1\nj1939", "AccelPedalPos2\nj1939", "ActMaxAvailEngPercentTorque\nj1939", "EEC2.EngPercentLoadAtCurrentSpeed\nj1939", "RemoteAccelPedalPos\nj1939", "RoadSpeedLimitStatus\nj1939", "VhclAccelerationRateLimitStatus\nj1939"]}, {"XNET Frame"="EEC3\nj1939", "Signals"=["AftrTrtmntExhustDewPointMessage\nj1939", "AftrTrtmntIntakeDewPointMessage\nj1939", "EngsDesiredOperatingSpeed\nj1939", "EngsDsrdOprtngSpdAsymmtryAdjstmn\nj1939", "EstEngPrsticLossesPercentTorque\nj1939", "ExhaustGasMass\nj1939", "NominalFrictionPercentTorque\nj1939"]}, {"XNET Frame"="EEC4\nj1939", "Signals"=["CrnkAttmptCntOnPrsntStrtAttempt\nj1939", "EngRatedPower\nj1939", "EngRatedSpeed\nj1939", "EngRotationDirection\nj1939"]}, {"XNET Frame"="EEC5\nj1939", "Signals"=["EngExhstGsRcirculationValveCtrl\nj1939", "EngTrb1ClclatedTurbineInletTemp\nj1939", "EngTrb1ClcltedTurbineOutletTemp\nj1939", "EngVrblGmtryTrbArCtrlShtffValve\nj1939", "EngVrblGometryTurbo1ActuatorPos\nj1939"]}, {"XNET Frame"="EEC6\nj1939", "Signals"=["EngTrbCmprssorBypassActuatorPos\nj1939", "EngTurboCompressorCtrl\nj1939", "EngVrableGeometryTurboActuator1\nj1939"]}, {"XNET Frame"="EEC7\nj1939", "Signals"=["EngExhstGsRcirculationValve2Pos\nj1939", "EngExhstGsRecirculationValvePos\nj1939"]}, {"XNET Frame"="EEC8\nj1939", "Signals"=["EngExhstGsRcrculationValve2Ctrl\nj1939"]}, {"XNET Frame"="EES\nj1939", "Signals"=["ElectricalLoad\nj1939", "SafetyWireStatus\nj1939", "TurningGearEngaged\nj1939"]}, {"XNET Frame"="EFL_P1\nj1939", "Signals"=["EngCoolantLevel\nj1939", "EngCoolantPress\nj1939", "EngCrankcasePress\nj1939", "EngExCrankcaseBlowbyPress\nj1939", "EngFuelDeliveryPress\nj1939", "EngOilLevel\nj1939", "EngOilPress\nj1939"]}, {"XNET Frame"="EFL_P2\nj1939", "Signals"=["EngInjectionCtrlPress\nj1939", "EngInjectorMeteringRail1Press\nj1939", "EngInjectorMeteringRail2Press\nj1939", "EngInjectorTimingRail1Press\nj1939"]}, {"XNET Frame"="EFL_P3\nj1939", "Signals"=["EngExhstGsRcrculationInletPress\nj1939", "EngIntkVlvActtionSystemOilPress\nj1939"]}, {"XNET Frame"="EFL_P4\nj1939", "Signals"=["EngAftercoolerCoolantLevel\nj1939", "EngCentrifugalOilFilterSpeed\nj1939", "EngChargeAirCooler1InletPress\nj1939", "EngChargeAirCooler2InletPress\nj1939", "EngChargeAirCoolerOutletPress\nj1939", "EngCoolantPumpDiffPress\nj1939", "EngIntercoolerCoolantLevel\nj1939"]}, {"XNET Frame"="EFL_P5\nj1939", "Signals"=["EngIntkVlvActtonOilPressForCyl1\nj1939", "EngIntkVlvActtonOilPressForCyl2\nj1939", "EngIntkVlvActtonOilPressForCyl3\nj1939", "EngIntkVlvActtonOilPressForCyl4\nj1939"]}, {"XNET Frame"="EFL_P6\nj1939", "Signals"=["EngIntkVlvActtonOilPressForCyl5\nj1939", "EngIntkVlvActtonOilPressForCyl6\nj1939", "EngIntkVlvActtonOilPressForCyl7\nj1939", "EngIntkVlvActtonOilPressForCyl8\nj1939"]}, {"XNET Frame"="EFL_P7\nj1939", "Signals"=["EngIntkVlvActtnOilPressForCyl10\nj1939", "EngIntkVlvActtnOilPressForCyl11\nj1939", "EngIntkVlvActtnOilPressForCyl12\nj1939", "EngIntkVlvActtonOilPressForCyl9\nj1939"]}, {"XNET Frame"="EFL_P8\nj1939", "Signals"=["EngIntkVlvActtnOilPressForCyl13\nj1939", "EngIntkVlvActtnOilPressForCyl14\nj1939", "EngIntkVlvActtnOilPressForCyl15\nj1939", "EngIntkVlvActtnOilPressForCyl16\nj1939"]}, {"XNET Frame"="EFL_P9\nj1939", "Signals"=["EngIntkVlvActtnOilPressForCyl17\nj1939", "EngIntkVlvActtnOilPressForCyl18\nj1939", "EngIntkVlvActtnOilPressForCyl19\nj1939", "EngIntkVlvActtnOilPressForCyl20\nj1939"]}, {"XNET Frame"="EFS\nj1939", "Signals"=["EngCoolantPreheatedState\nj1939", "EngFuelFilterSucSideDiffPress\nj1939", "EngFuelSupplyPumpInletPress\nj1939", "EngOilFilterOutletPress\nj1939", "EngOilLevelRemoteReservoir\nj1939", "EngOilPreHeatedState\nj1939", "EngOilPrimingPumpSwitch\nj1939", "EngOilPrimingState\nj1939", "EngVentilationStatus\nj1939", "EngWasteOilReservoirLevel\nj1939"]}, {"XNET Frame"="EGF1\nj1939", "Signals"=["EngExhstGsRcrcltionMassFlowRate\nj1939", "EngInletAirMassFlowRate\nj1939"]}, {"XNET Frame"="EGRBV\nj1939", "Signals"=["EGRCoolerBypassActuatorPostion\nj1939"]}, {"XNET Frame"="EH\nj1939", "Signals"=["TotalECUDistance\nj1939", "TotalECURunTime\nj1939"]}, {"XNET Frame"="EI\nj1939", "Signals"=["EngExhaustGasPress\nj1939", "EngFuelRackPos\nj1939", "EngMassFlow\nj1939", "EngPrefilterOilPress\nj1939", "InstantaneousEstBrakePower\nj1939"]}, {"XNET Frame"="EJM1\nj1939", "Signals"=["Joystick1GripXAxisPos\nj1939", "Joystick1GripYAxisPos\nj1939", "Joystick1ThetaAxisPos\nj1939", "Jystck1GripXAxisDetentPosStatus\nj1939", "Jystck1GripYAxisDetentPosStatus\nj1939", "Jystck1GrpXAxisNeutralPosStatus\nj1939", "Jystck1GrpXAxsLvrLftNgtvPsSttus\nj1939", "Jystck1GrpXAxsLvrRghtPstvPsStts\nj1939", "Jystck1GrpYAxisNeutralPosStatus\nj1939", "Jystck1GrpYAxsLvrBckNgtvPsSttus\nj1939", "Jystck1GrpYAxsLvrFrwrdPstvPsStts\nj1939", "Jystck1ThetaAxisDetentPosStatus\nj1939", "Jystck1ThtAxsClckwsPstvPsStatus\nj1939", "Jystck1ThtAxsCntrClckwsNgtvPsStt\nj1939", "Jystck1ThtaAxisNeutralPosStatus\nj1939"]}, {"XNET Frame"="EJM2\nj1939", "Signals"=["Joystick2GripXAxisPos\nj1939", "Joystick2GripYAxisPos\nj1939", "Joystick2ThetaAxisPos\nj1939", "Jystck2GripXAxisDetentPosStatus\nj1939", "Jystck2GripYAxisDetentPosStatus\nj1939", "Jystck2GrpXAxisNeutralPosStatus\nj1939", "Jystck2GrpXAxsLvrLftNgtvPsSttus\nj1939", "Jystck2GrpXAxsLvrRghtPstvPsStts\nj1939", "Jystck2GrpYAxisNeutralPosStatus\nj1939", "Jystck2GrpYAxsLvrBckNgtvPsSttus\nj1939", "Jystck2GrpYAxsLvrFrwrdPstvPsStts\nj1939", "Jystck2ThetaAxisDetentPosStatus\nj1939", "Jystck2ThtAxsClckwsPstvPsStatus\nj1939", "Jystck2ThtAxsCntrClckwsNgtvPsStt\nj1939", "Jystck2ThtaAxisNeutralPosStatus\nj1939"]}, {"XNET Frame"="EJM3\nj1939", "Signals"=["Joystick3GripXAxisPos\nj1939", "Joystick3GripYAxisPos\nj1939", "Joystick3ThetaAxisPos\nj1939", "Jystck3GripXAxisDetentPosStatus\nj1939", "Jystck3GripYAxisDetentPosStatus\nj1939", "Jystck3GrpXAxisNeutralPosStatus\nj1939", "Jystck3GrpXAxsLvrLftNgtvPsSttus\nj1939", "Jystck3GrpXAxsLvrRghtPstvPsStts\nj1939", "Jystck3GrpYAxisNeutralPosStatus\nj1939", "Jystck3GrpYAxsLvrBckNgtvPsSttus\nj1939", "Jystck3GrpYAxsLvrFrwrdPstvPsStts\nj1939", "Jystck3ThetaAxisDetentPosStatus\nj1939", "Jystck3ThtAxsClckwsPstvPsStatus\nj1939", "Jystck3ThtAxsCntrClckwsNgtvPsStt\nj1939", "Jystck3ThtaAxisNeutralPosStatus\nj1939"]}, {"XNET Frame"="EO1\nj1939", "Signals"=["EngActualExhaustOxygen\nj1939", "EngDesiredExhaustOxygen\nj1939", "EngDesiredRatedExhaustOxygen\nj1939", "EngExhstGsOxygnSnsrClsdLpOprton\nj1939", "EngExhstGsOxygnSnsrFlngCrrction\nj1939"]}, {"XNET Frame"="EOAC\nj1939", "Signals"=["TravelVelocityCtrlPos\nj1939"]}, {"XNET Frame"="EP\nj1939", "Signals"=["DataMemoryUsage\nj1939", "KeepAliveBatteryConsumption\nj1939"]}, {"XNET Frame"="EPD\nj1939", "Signals"=["PayloadPercentage\nj1939"]}, {"XNET Frame"="EPT1\nj1939", "Signals"=["EngExhaustGasPort1Temp\nj1939", "EngExhaustGasPort2Temp\nj1939", "EngExhaustGasPort3Temp\nj1939", "EngExhaustGasPort4Temp\nj1939"]}, {"XNET Frame"="EPT2\nj1939", "Signals"=["EngExhaustGasPort5Temp\nj1939", "EngExhaustGasPort6Temp\nj1939", "EngExhaustGasPort7Temp\nj1939", "EngExhaustGasPort8Temp\nj1939"]}, {"XNET Frame"="EPT3\nj1939", "Signals"=["EngExhaustGasPort10Temp\nj1939", "EngExhaustGasPort11Temp\nj1939", "EngExhaustGasPort12Temp\nj1939", "EngExhaustGasPort9Temp\nj1939"]}, {"XNET Frame"="EPT4\nj1939", "Signals"=["EngExhaustGasPort13Temp\nj1939", "EngExhaustGasPort14Temp\nj1939", "EngExhaustGasPort15Temp\nj1939", "EngExhaustGasPort16Temp\nj1939"]}, {"XNET Frame"="EPT5\nj1939", "Signals"=["EngExhaustGasPort17Temp\nj1939", "EngExhaustGasPort18Temp\nj1939", "EngExhaustGasPort19Temp\nj1939", "EngExhaustGasPort20Temp\nj1939"]}, {"XNET Frame"="ERC1\nj1939", "Signals"=["ActlMxAvlblRtarderPercentTorque\nj1939", "ActualRetarderPercentTorque\nj1939", "DrvrsDmandRetarderPercentTorque\nj1939", "EngCoolantLoadIncrease\nj1939", "IntendedRetarderPercentTorque\nj1939", "RetarderEnableBrakeAssistSwitch\nj1939", "RetarderEnableShiftAssistSwitch\nj1939", "RetarderRqingBrakeLight\nj1939", "RetarderSelectionNonEng\nj1939", "RetarderTorqueMode\nj1939", "SrcAddrssOfCtrllngDvcFrRtrdrCtrl\nj1939"]}, {"XNET Frame"="ERC2\nj1939", "Signals"=["TransOutputRetarder\nj1939"]}, {"XNET Frame"="ESC1\nj1939", "Signals"=["ActualInnerWheelSteerAngle\nj1939", "ESC1.AxleLocation\nj1939", "StatusOfSteerAxle\nj1939", "SteerType\nj1939", "SterableLiftAxleLoweringInhibit\nj1939", "TypeOfSteerForces\nj1939", "TypeOfSteerTrans\nj1939"]}, {"XNET Frame"="ESV1\nj1939", "Signals"=["EngSparkPlug1\nj1939", "EngSparkPlug2\nj1939", "EngSparkPlug3\nj1939", "EngSparkPlug4\nj1939"]}, {"XNET Frame"="ESV2\nj1939", "Signals"=["EngSparkPlug5\nj1939", "EngSparkPlug6\nj1939", "EngSparkPlug7\nj1939", "EngSparkPlug8\nj1939"]}, {"XNET Frame"="ESV3\nj1939", "Signals"=["EngSparkPlug10\nj1939", "EngSparkPlug11\nj1939", "EngSparkPlug12\nj1939", "EngSparkPlug9\nj1939"]}, {"XNET Frame"="ESV4\nj1939", "Signals"=["EngSparkPlug13\nj1939", "EngSparkPlug14\nj1939", "EngSparkPlug15\nj1939", "EngSparkPlug16\nj1939"]}, {"XNET Frame"="ESV5\nj1939", "Signals"=["EngSparkPlug17\nj1939", "EngSparkPlug18\nj1939", "EngSparkPlug19\nj1939", "EngSparkPlug20\nj1939"]}, {"XNET Frame"="ESV6\nj1939", "Signals"=["EngSparkPlug21\nj1939", "EngSparkPlug22\nj1939", "EngSparkPlug23\nj1939", "EngSparkPlug24\nj1939"]}, {"XNET Frame"="ET\nj1939", "Signals"=["EngExhstExhstGsTempLeftManifold\nj1939", "EngExhstExhstGsTmpRightManifold\nj1939"]}, {"XNET Frame"="ET1\nj1939", "Signals"=["EngCoolantTemp\nj1939", "EngFuelTemp\nj1939", "EngIntercoolerTemp\nj1939", "EngIntercoolerThermostatOpening\nj1939", "EngOilTemp1\nj1939", "EngTurboOilTemp\nj1939"]}, {"XNET Frame"="ET2\nj1939", "Signals"=["EngECUTemp\nj1939", "EngExhaustGasRecirculationTemp\nj1939", "EngExhstGsRcirculationDiffPress\nj1939", "EngOilTemp2\nj1939"]}, {"XNET Frame"="ET3\nj1939", "Signals"=["EngChargeAirCoolerOutletTemp\nj1939", "EngCoolantTempHiRes\nj1939", "EngIntakeManifold1AirTemp\nj1939", "EngIntkVlvActationSystemOilTemp\nj1939"]}, {"XNET Frame"="ETC1\nj1939", "Signals"=["EngMomentaryOverspeedEnable\nj1939", "ETC1.PercentClutchSlip\nj1939", "ProgressiveShiftDisable\nj1939", "SrcAddrssOfCtrllngDvcFrTrnsCtrl\nj1939", "TorqueConverterLockupEngaged\nj1939", "TransDrivelineEngaged\nj1939", "TransInputShaftSpeed\nj1939", "TransOutputShaftSpeed\nj1939", "TransShiftInProcess\nj1939"]}, {"XNET Frame"="ETC2\nj1939", "Signals"=["TransActualGearRatio\nj1939", "TransCurrentGear\nj1939", "TransCurrentRange\nj1939", "TransRqedRange\nj1939", "TransSelectedGear\nj1939"]}, {"XNET Frame"="ETC3\nj1939", "Signals"=["TransClutchActuator\nj1939", "TransDefuelActuator\nj1939", "TransInertiaBrakeActuator\nj1939", "TransLockupClutchActuator\nj1939", "TransRangeHighActuator\nj1939", "TransRangeLowActuator\nj1939", "TransShiftFingerGearActuator1\nj1939", "TransShiftFingerGearActuator2\nj1939", "TransShiftFingerGearPos\nj1939", "TransShiftFingerRailActuator1\nj1939", "TransShiftFingerRailActuator2\nj1939", "TransShiftFingerRailPos\nj1939", "TransSplitterDirectActuator\nj1939", "TransSplitterIndirectActuator\nj1939", "TrnsShftFngrCenterRailIndicator\nj1939", "TrnsShftFngrEngagementIndicator\nj1939", "TrnsShiftFingerNeutralIndicator\nj1939"]}, {"XNET Frame"="ETC4\nj1939", "Signals"=["TransSynchronizerBrakeValue\nj1939", "TransSynchronizerClutchValue\nj1939"]}, {"XNET Frame"="ETC5\nj1939", "Signals"=["TransForwardDirectionSwitch\nj1939", "TransHighRangeSenseSwitch\nj1939", "TransLowRangeSenseSwitch\nj1939", "TransNeutralSwitch\nj1939", "TransReverseDirectionSwitch\nj1939"]}, {"XNET Frame"="ETC6\nj1939", "Signals"=["ClutchLifeRemaining\nj1939", "HighestPossibleGear\nj1939", "LowestPossibleGear\nj1939", "RecommendedGear\nj1939"]}, {"XNET Frame"="ETC7\nj1939", "Signals"=["ActiveShiftConsoleIndicator\nj1939", "TransEngCrankEnable\nj1939", "TransMode1Indicator\nj1939", "TransMode2Indicator\nj1939", "TransMode3Indicator\nj1939", "TransMode4Indicator\nj1939", "TransReadyForBrakeRelease\nj1939", "TransRqedGearFeedback\nj1939", "TransRqedRangeDisplayBlankState\nj1939", "TransRqedRangeDisplayFlashState\nj1939", "TransShiftInhibitIndicator\nj1939"]}, {"XNET Frame"="ETC8\nj1939", "Signals"=["TransTorqueConverterRatio\nj1939"]}, {"XNET Frame"="FD\nj1939", "Signals"=["EstPercentFanSpeed\nj1939", "FanDriveState\nj1939", "FanSpeed\nj1939"]}, {"XNET Frame"="FL\nj1939", "Signals"=["EngFuelLeakage1\nj1939", "EngFuelLeakage2\nj1939"]}, {"XNET Frame"="FLI1\nj1939", "Signals"=["LaneDepartureImminentLeftSide\nj1939", "LaneDepartureImminentRightSide\nj1939"]}, {"XNET Frame"="FLI2\nj1939", "Signals"=["LaneTrackingStatusLeftSide\nj1939", "LaneTrackingStatusRightSide\nj1939", "LnDprtureIndicationEnableStatus\nj1939"]}, {"XNET Frame"="FLIC\nj1939", "Signals"=["LaneDepartureWarningEnableCmd\nj1939"]}, {"XNET Frame"="FMS\nj1939", "Signals"=["FMSstandardDiagnosticsSupported\nj1939", "FMSstandardRqsSupported\nj1939", "FMSstandardSWversionSupported\nj1939"]}, {"XNET Frame"="FWD\nj1939", "Signals"=["FrontWheelDriveActuatorStatus\nj1939"]}, {"XNET Frame"="FWSS1\nj1939", "Signals"=["FifthWheelDrawbarForce\nj1939", "FifthWheelRollMoment\nj1939", "FifthWheelRollWarningIndicator\nj1939", "FifthWheelVerticalForce\nj1939"]}, {"XNET Frame"="FWSS2\nj1939", "Signals"=["FfthWhlLckCoupleStatusIndicator\nj1939", "FfthWhlLckRadyToCoupleIndicator\nj1939", "FifthWheelErrorStatus\nj1939", "FifthWheelSliderLockIndicator\nj1939", "FifthWheelSliderPos\nj1939"]}, {"XNET Frame"="GAAC\nj1939", "Signals"=["GeneratorAverageACFrequency\nj1939", "GeneratorAverageACRMSCurrent\nj1939", "GnrtrAvrageLineLineACRMSVoltage\nj1939", "GnrtrAvrgLneNeutralACRMSVoltage\nj1939"]}, {"XNET Frame"="GFC\nj1939", "Signals"=["TotalFuelUsed\nj1939", "TripFuel\nj1939"]}, {"XNET Frame"="GFD\nj1939", "Signals"=["SpecificHeatRatio\nj1939"]}, {"XNET Frame"="GFI1\nj1939", "Signals"=["EngFuelSpecificGravity\nj1939", "GFI1.TotalEngPTOFuelUsed\nj1939", "GFI1.TripAverageFuelRate\nj1939"]}, {"XNET Frame"="GFI2\nj1939", "Signals"=["EngFuelFlowRate1\nj1939", "EngFuelFlowRate2\nj1939", "EngFuelValve1Pos\nj1939", "EngFuelValve2Pos\nj1939", "EngRqedFuelValve1Pos\nj1939", "EngRqedFuelValve2Pos\nj1939"]}, {"XNET Frame"="GFI3\nj1939", "Signals"=["EngFuelTemp2\nj1939", "EngFuelValve2InletAbsPress\nj1939", "EngFuelValve2OutletAbsPress\nj1939", "EngGasMassFlowRate2\nj1939"]}, {"XNET Frame"="GFP\nj1939", "Signals"=["EngAirToFuelDiffPress\nj1939", "EngFuelValve1OutletAbsPress\nj1939", "EngFuelValveDiffPress\nj1939", "EngFuelValveInletAbsPress\nj1939"]}, {"XNET Frame"="GPAAC\nj1939", "Signals"=["GeneratorPhaseAACFrequency\nj1939", "GeneratorPhaseAACRMSCurrent\nj1939", "GnrtrPhsALneNeutralACRMSVoltage\nj1939", "GnrtrPhseABLineLineACRMSVoltage\nj1939"]}, {"XNET Frame"="GPAACP\nj1939", "Signals"=["GeneratorPhaseAApparentPower\nj1939", "GeneratorPhaseARealPower\nj1939"]}, {"XNET Frame"="GPAACR\nj1939", "Signals"=["GeneratorPhaseAPowerFactor\nj1939", "GeneratorPhaseAReactivePower\nj1939", "GnratorPhaseAPowerFactorLagging\nj1939"]}, {"XNET Frame"="GPBAC\nj1939", "Signals"=["GeneratorPhaseBACFrequency\nj1939", "GeneratorPhaseBACRMSCurrent\nj1939", "GnrtrPhsBLneNeutralACRMSVoltage\nj1939", "GnrtrPhseBCLineLineACRMSVoltage\nj1939"]}, {"XNET Frame"="GPBACP\nj1939", "Signals"=["GeneratorPhaseBApparentPower\nj1939", "GeneratorPhaseBRealPower\nj1939"]}, {"XNET Frame"="GPBACRP\nj1939", "Signals"=["GeneratorPhaseBPowerFactor\nj1939", "GeneratorPhaseBReactivePower\nj1939", "GnratorPhaseBPowerFactorLagging\nj1939"]}, {"XNET Frame"="GPCAC\nj1939", "Signals"=["GeneratorPhaseCACFrequency\nj1939", "GeneratorPhaseCACRMSCurrent\nj1939", "GnrtrPhsCLneNeutralACRMSVoltage\nj1939", "GnrtrPhseCALineLineACRMSVoltage\nj1939"]}, {"XNET Frame"="GPCACP\nj1939", "Signals"=["GeneratorPhaseCApparentPower\nj1939", "GeneratorPhaseCRealPower\nj1939"]}, {"XNET Frame"="GPCACR\nj1939", "Signals"=["GeneratorPhaseCPowerFactor\nj1939", "GeneratorPhaseCReactivePower\nj1939", "GnratorPhaseCPowerFactorLagging\nj1939"]}, {"XNET Frame"="GPM11\nj1939", "Signals"=["AntiTheftDeviceReq\nj1939", "ODDRequest\nj1939", "GPM11.VehicleType\nj1939"]}, {"XNET Frame"="GPM12\nj1939", "Signals"=["EngineSpeedLowerLimit\nj1939", "EngineSpeedUpperLimit\nj1939", "GPM12.MaxVehicleSpeedLimit\nj1939"]}, {"XNET Frame"="GPM13\nj1939", "Signals"=["ActualEngine_PercTorque\nj1939", "DriversDemandEngine_PercTorque\nj1939", "EngineControlAllowed\nj1939", "EngineRunning\nj1939", "EngineSpeed\nj1939", "EngineTorqueMode\nj1939", "PercentLoadAtCurrentSpeed\nj1939", "VehicleSpeed\nj1939"]}, {"XNET Frame"="GPM14\nj1939", "Signals"=["AccelPedalLowIdleSwitch\nj1939", "AccelPedalPosition\nj1939", "ClutchIndptdPTOFeedback\nj1939", "CurrentGear\nj1939", "FirstClutchDpdtPTOFeedback\nj1939", "FirstEngineMtdPTOFeedback\nj1939", "PTOControlAllowed\nj1939", "GPM14.PercentClutchSlip\nj1939", "SecClutchDptdPTOFeedback\nj1939", "SecEngineMtdPTOFeedback\nj1939", "StarterActive\nj1939", "TorqueConvOilTemp\nj1939", "TorqueConvtOilTempWarning\nj1939"]}, {"XNET Frame"="GPM15\nj1939", "Signals"=["EngineCoolantTempWarning\nj1939", "GPM15.EngineCoolantTemperature\nj1939", "EngineOilPressure\nj1939", "EngineOilPressureWarning\nj1939", "EngineOilTemperature\nj1939", "FuelLevelWarning\nj1939", "ReferenceEngineTorque\nj1939"]}, {"XNET Frame"="GPM16\nj1939", "Signals"=["AmbientAirTemperature\nj1939"]}, {"XNET Frame"="GPM21\nj1939", "Signals"=["GPM21.VehicleType\nj1939"]}, {"XNET Frame"="GPM22\nj1939", "Signals"=["AntiTheftDeviceStatus\nj1939", "BodyFluidLevel\nj1939", "BodyPressure\nj1939", "ODDStatus\nj1939", "RearObstacleDistance\nj1939", "ThermalBodyTemperature\nj1939"]}, {"XNET Frame"="GPM23\nj1939", "Signals"=["ReqEngineSpeed\nj1939", "ReqEngineSpeedLimit\nj1939", "ReqEngineSpeedLowerLim\nj1939", "ReqEngineSpeedUpperLim\nj1939", "ReqEngineTorqueLimit\nj1939"]}, {"XNET Frame"="GPM24\nj1939", "Signals"=["ClutchIndpdtPTOSwitch\nj1939", "EngineStartSwitch\nj1939", "EngineStopSwitch\nj1939", "FirstClutchDpdtPTOSwitch\nj1939", "FirstEngineMtdPTOSwitch\nj1939", "OperatingPanelActive\nj1939", "RefusePackerStepSwitch\nj1939", "RqstedPercentClutchSlip\nj1939", "SecClutchDpdtPTOSwitch\nj1939", "SecEngineMtdPTOSwitch\nj1939", "StarterLockoutSwitch\nj1939"]}, {"XNET Frame"="GPM25\nj1939", "Signals"=["TrailRightRearWidIndLight\nj1939", "TrailerInteriorLight\nj1939", "TrailerLeftCrnMarkerLight\nj1939", "TrailerLeftDirIndLight\nj1939", "TrailerLeftRearFogLight\nj1939", "TrailerLeftRearLight\nj1939", "TrailerLeftRearRegPltLight\nj1939", "TrailerLeftRearWidIndLight\nj1939", "TrailerLeftReversingLight\nj1939", "TrailerLeftSideMarkerLight\nj1939", "TrailerLeftStopLight\nj1939", "TrailerRearWarningLight\nj1939", "TrailerRightCrnMarkerLight\nj1939", "TrailerRightDirIndLight\nj1939", "TrailerRightRearFogLight\nj1939", "TrailerRightRearLight\nj1939", "TrailerRightRearRegPltLight\nj1939", "TrailerRightReversingLight\nj1939", "TrailerRightSideMrkLight\nj1939", "TrailerRightStopLight\nj1939", "TrailerRotatingIdentLight\nj1939", "TrailerWorkLamp\nj1939"]}, {"XNET Frame"="GTACE\nj1939", "Signals"=["GeneratorTotalKWHoursExport\nj1939", "GeneratorTotalKWHoursImport\nj1939"]}, {"XNET Frame"="GTACP\nj1939", "Signals"=["GeneratorTotalApparentPower\nj1939", "GeneratorTotalRealPower\nj1939"]}, {"XNET Frame"="GTACR\nj1939", "Signals"=["GeneratorOverallPowerFactor\nj1939", "GeneratorTotalReactivePower\nj1939", "GnrtorOverallPowerFactorLagging\nj1939"]}, {"XNET Frame"="HBS\nj1939", "Signals"=["HydBrakeFluidLevelSwitch\nj1939", "HydBrakePressCircuit1\nj1939", "HydBrakePressCircuit2\nj1939", "HydBrakeSystemAudibleWarningCmd\nj1939", "HydBrkPressWarningStateCircuit1\nj1939", "HydBrkPressWarningStateCircuit2\nj1939", "HydBrkePressSupplyStateCircuit1\nj1939", "HydBrkePressSupplyStateCircuit2\nj1939"]}, {"XNET Frame"="HOURS\nj1939", "Signals"=["EngTotalHoursOfOperation\nj1939", "EngTotalRevolutions\nj1939"]}, {"XNET Frame"="HPG\nj1939", "Signals"=["EngHydPressGovernorSwitch\nj1939", "EngHydPrssGovernorModeIndicator\nj1939", "FireApparatusPumpEngagement\nj1939", "HydPress\nj1939"]}, {"XNET Frame"="HRW\nj1939", "Signals"=["FrontAxleLeftWheelSpeed\nj1939", "FrontAxleRightWheelSpeed\nj1939", "RearAxleLeftWheelSpeed\nj1939", "RearAxleRightWheelSpeed\nj1939"]}, {"XNET Frame"="HTR\nj1939", "Signals"=["AuxHeaterInputAirTemp\nj1939", "AuxHeaterMode\nj1939", "AuxHeaterOutputCoolantTemp\nj1939", "AuxHeaterOutputPowerPercent\nj1939", "AuxilaryHeaterWaterPumpStatus\nj1939", "CabHeatingZone\nj1939", "CabVentilation\nj1939", "EngHeatingZone\nj1939"]}, {"XNET Frame"="IC1\nj1939", "Signals"=["EngAirFilter1DiffPress\nj1939", "EngAirInletPress\nj1939", "EngCoolantFilterDiffPress\nj1939", "EngExhaustGasTemp\nj1939", "EngIntakeManifold1Temp\nj1939", "EngParticulateTrapInletPress\nj1939", "IC1.EngTurboBoostPress\nj1939"]}, {"XNET Frame"="IC2\nj1939", "Signals"=["EngAirFilter2DiffPress\nj1939", "EngAirFilter3DiffPress\nj1939", "EngAirFilter4DiffPress\nj1939", "EngIntakeManifold1AbsPress\nj1939", "EngIntakeManifold2Press\nj1939"]}, {"XNET Frame"="IMT1\nj1939", "Signals"=["EngTurbo1BoostPress\nj1939", "EngTurbo2BoostPress\nj1939", "EngTurbo3BoostPress\nj1939", "EngTurbo4BoostPress\nj1939"]}, {"XNET Frame"="IMT2\nj1939", "Signals"=["EngIntakeManifold2Temp\nj1939", "EngIntakeManifold3Temp\nj1939", "EngIntakeManifold4Temp\nj1939", "EngIntakeManifold5Temp\nj1939", "EngIntakeManifold6Temp\nj1939"]}, {"XNET Frame"="IO\nj1939", "Signals"=["EngTotalIdleFuelUsed\nj1939", "EngTotalIdleHours\nj1939"]}, {"XNET Frame"="ISC\nj1939", "Signals"=["EngOprtrPrmryIntrmdtSpeedSelect\nj1939"]}, {"XNET Frame"="ISCS\nj1939", "Signals"=["EngOprtrPrmryIntrmdtSpdSlctStte\nj1939"]}, {"XNET Frame"="ISO1\nj1939", "Signals"=["EngCyl1IgntTransSecondOutput\nj1939", "EngCyl2IgntTransSecondOutput\nj1939", "EngCyl3IgntTransSecondOutput\nj1939", "EngCyl4IgntTransSecondOutput\nj1939", "EngCyl5IgntTransSecondOutput\nj1939", "EngCyl6IgntTransSecondOutput\nj1939", "EngCyl7IgntTransSecondOutput\nj1939", "EngCyl8IgntTransSecondOutput\nj1939"]}, {"XNET Frame"="ISO15765_Funct\nj1939", "Signals"=["ISO15765_Funct.BlockSize\nj1939", "ISO15765_Funct.FirstFrameDataLength\nj1939", "ISO15765_Funct.FlowStatus\nj1939", "ISO15765_Funct.ProtocolCtrlInformation\nj1939", "ISO15765_Funct.SN\nj1939", "ISO15765_Funct.SeparationTime\nj1939", "ISO15765_Funct.SingleFrameDataLength\nj1939"]}, {"XNET Frame"="ISO15765_Phys\nj1939", "Signals"=["ISO15765_Phys.BlockSize\nj1939", "ISO15765_Phys.FirstFrameDataLength\nj1939", "ISO15765_Phys.FlowStatus\nj1939", "ISO15765_Phys.ProtocolCtrlInformation\nj1939", "ISO15765_Phys.SN\nj1939", "ISO15765_Phys.SeparationTime\nj1939", "ISO15765_Phys.SingleFrameDataLength\nj1939"]}, {"XNET Frame"="ISO2\nj1939", "Signals"=["EngCyl10IgntTransSecondOutput\nj1939", "EngCyl11IgntTransSecondOutput\nj1939", "EngCyl12IgntTransSecondOutput\nj1939", "EngCyl13IgntTransSecondOutput\nj1939", "EngCyl14IgntTransSecondOutput\nj1939", "EngCyl15IgntTransSecondOutput\nj1939", "EngCyl16IgntTransSecondOutput\nj1939", "EngCyl9IgntTransSecondOutput\nj1939"]}, {"XNET Frame"="ISO3\nj1939", "Signals"=["EngCyl17IgntTransSecondOutput\nj1939", "EngCyl18IgntTransSecondOutput\nj1939", "EngCyl19IgntTransSecondOutput\nj1939", "EngCyl20IgntTransSecondOutput\nj1939"]}, {"XNET Frame"="IT1\nj1939", "Signals"=["EngCyl1IgntTiming\nj1939", "EngCyl2IgntTiming\nj1939", "EngCyl3IgntTiming\nj1939", "EngCyl4IgntTiming\nj1939"]}, {"XNET Frame"="IT2\nj1939", "Signals"=["EngCyl5IgntTiming\nj1939", "EngCyl6IgntTiming\nj1939", "EngCyl7IgntTiming\nj1939", "EngCyl8IgntTiming\nj1939"]}, {"XNET Frame"="IT3\nj1939", "Signals"=["EngCyl10IgntTiming\nj1939", "EngCyl11IgntTiming\nj1939", "EngCyl12IgntTiming\nj1939", "EngCyl9IgntTiming\nj1939"]}, {"XNET Frame"="IT4\nj1939", "Signals"=["EngCyl13IgntTiming\nj1939", "EngCyl14IgntTiming\nj1939", "EngCyl15IgntTiming\nj1939", "EngCyl16IgntTiming\nj1939"]}, {"XNET Frame"="IT5\nj1939", "Signals"=["EngCyl17IgntTiming\nj1939", "EngCyl18IgntTiming\nj1939", "EngCyl19IgntTiming\nj1939", "EngCyl20IgntTiming\nj1939"]}, {"XNET Frame"="IT6\nj1939", "Signals"=["EngActualIgntTiming\nj1939", "EngDesiredIgntTiming1\nj1939", "EngDesiredIgntTiming2\nj1939", "EngDesiredIgntTiming3\nj1939"]}, {"XNET Frame"="J2012\nj1939", "Signals"=["J2012DTCOccurrenceCount\nj1939", "J2012DTCStatus\nj1939", "NumberOfJ2012DTCs\nj1939"]}, {"XNET Frame"="KL1\nj1939", "Signals"=["EngCyl1KnockLevel\nj1939", "EngCyl2KnockLevel\nj1939", "EngCyl3KnockLevel\nj1939", "EngCyl4KnockLevel\nj1939", "EngCyl5KnockLevel\nj1939", "EngCyl6KnockLevel\nj1939", "EngCyl7KnockLevel\nj1939", "EngCyl8KnockLevel\nj1939"]}, {"XNET Frame"="KL2\nj1939", "Signals"=["EngCyl10KnockLevel\nj1939", "EngCyl11KnockLevel\nj1939", "EngCyl12KnockLevel\nj1939", "EngCyl13KnockLevel\nj1939", "EngCyl14KnockLevel\nj1939", "EngCyl15KnockLevel\nj1939", "EngCyl16KnockLevel\nj1939", "EngCyl9KnockLevel\nj1939"]}, {"XNET Frame"="KL3\nj1939", "Signals"=["EngCyl17KnockLevel\nj1939", "EngCyl18KnockLevel\nj1939", "EngCyl19KnockLevel\nj1939", "EngCyl20KnockLevel\nj1939", "EngCyl21KnockLevel\nj1939", "EngCyl22KnockLevel\nj1939", "EngCyl23KnockLevel\nj1939", "EngCyl24KnockLevel\nj1939"]}, {"XNET Frame"="LBC\nj1939", "Signals"=["BladeCtrlMode\nj1939", "BladeDurationAndDirection\nj1939"]}, {"XNET Frame"="LC\nj1939", "Signals"=["AltBeamHeadLightCmd\nj1939", "BackUpLightAndAlarmHornCmd\nj1939", "CenterStopLightCmd\nj1939", "HighBeamHeadLightCmd\nj1939", "ImplementClearanceLightCmd\nj1939", "ImplementLeftFacingWorkLightCmd\nj1939", "ImplementMarkerLightCmd\nj1939", "ImplementOEMOption1LightCmd\nj1939", "ImplementOEMOption2LightCmd\nj1939", "ImplementRearWorkLightCmd\nj1939", "ImplmentLeftForwardWorkLightCmd\nj1939", "ImplmentRightFacingWorkLightCmd\nj1939", "ImplmntRightForwardWorkLightCmd\nj1939", "LeftStopLightCmd\nj1939", "LeftTurnSignalLightsCmd\nj1939", "LightingDataRqCmd\nj1939", "LowBeamHeadLightCmd\nj1939", "RearFogLightCmd\nj1939", "RightStopLightCmd\nj1939", "RightTurnSignalLightsCmd\nj1939", "RotatingBeaconLightCmd\nj1939", "RunningLightCmd\nj1939", "TractorClearanceLightCmd\nj1939", "TractorFrontFogLightsCmd\nj1939", "TractorMarkerLightCmd\nj1939", "TrctrFrntHghMuntedWorkLightsCmd\nj1939", "TrctrFrntLwMountedWorkLightsCmd\nj1939", "TrctrRarLowMountedWorkLightsCmd\nj1939", "TrctrRrHighMountedWorkLightsCmd\nj1939", "TrctrSdHighMountedWorkLightsCmd\nj1939", "TrctrSdeLowMountedWorkLightsCmd\nj1939", "TrctrUndrsdMountedWorkLightsCmd\nj1939"]}, {"XNET Frame"="LD\nj1939", "Signals"=["AltBeamHeadLightData\nj1939", "BackUpLightAndAlarmHorn\nj1939", "CenterStopLight\nj1939", "HighBeamHeadLightData\nj1939", "ImplementClearanceLight\nj1939", "ImplementLeftFacingWorkLight\nj1939", "ImplementLeftForwardWorkLight\nj1939", "ImplementMarkerLight\nj1939", "ImplementOEMOption1Light\nj1939", "ImplementOEMOption2Light\nj1939", "ImplementRearWorkLight\nj1939", "ImplementRightFacingWorkLight\nj1939", "ImplementRightForwardWorkLight\nj1939", "LeftStopLight\nj1939", "LeftTurnSignalLights\nj1939", "LowBeamHeadLightData\nj1939", "RearFogLights\nj1939", "RightStopLight\nj1939", "RightTurnSignalLights\nj1939", "RotatingBeaconLight\nj1939", "RunningLight\nj1939", "TractorClearanceLight\nj1939", "TractorFrontFogLights\nj1939", "TractorMarkerLight\nj1939", "TractorRearLowMountedWorkLights\nj1939", "TractorSideLowMountedWorkLights\nj1939", "TrctorFrontLowMountedWorkLights\nj1939", "TrctorRearHighMountedWorkLights\nj1939", "TrctorSideHighMountedWorkLights\nj1939", "TrctrFrontHighMountedWorkLights\nj1939", "TrctrUndersideMountedWorkLights\nj1939"]}, {"XNET Frame"="LFC\nj1939", "Signals"=["EngTotalFuelUsed\nj1939", "EngTripFuel\nj1939"]}, {"XNET Frame"="LFE\nj1939", "Signals"=["EngAverageFuelEconomy\nj1939", "EngFuelRate\nj1939", "EngInstantaneousFuelEconomy\nj1939", "EngThrottle2Pos\nj1939", "EngThrottlePos\nj1939"]}, {"XNET Frame"="LFI\nj1939", "Signals"=["LFI.TotalEngPTOFuelUsed\nj1939", "LFI.TripAverageFuelRate\nj1939"]}]
  in  "Incoming Frames":T1[](array[typedef])=[{"XNET Frame"="A1\nj1939", "Signals"=["EngBlowerBypassValvePos\nj1939", "EngGasSupplyPress\nj1939"]}, {"XNET Frame"="AAC1\nj1939", "Signals"=["Aftertreatment1AirPressCtrl\nj1939", "Aftertreatment1AirSystemRelay\nj1939", "Aftertreatment1PurgeAirActuator\nj1939", "Aftertreatment1PurgeAirPress\nj1939", "Aftertreatment1SupplyAirPress\nj1939", "Aftrtreatment1AirEnableActuator\nj1939", "Aftrtrtment1AirPressActuatorPos\nj1939", "Aftrtrtmnt1AtmzationAirActuator\nj1939"]}, {"XNET Frame"="AAC2\nj1939", "Signals"=["Aftertreatment2AirPressCtrl\nj1939", "Aftertreatment2AirSystemRelay\nj1939", "Aftertreatment2PurgeAirActuator\nj1939", "Aftertreatment2PurgeAirPress\nj1939", "Aftertreatment2SupplyAirPress\nj1939", "Aftrtreatment2AirEnableActuator\nj1939", "Aftrtrtment2AirPressActuatorPos\nj1939", "Aftrtrtmnt2AtmzationAirActuator\nj1939"]}, {"XNET Frame"="AAC3\nj1939", "Signals"=["Aftertreatment1SecondAirPress\nj1939", "Aftertreatment1SecondAirTemp\nj1939", "Aftrtratment1SecondAirDiffPress\nj1939", "Aftrtreatment1SecondAirMassFlow\nj1939"]}, {"XNET Frame"="AAC4\nj1939", "Signals"=["Aftertreatment2SecondAirPress\nj1939", "Aftertreatment2SecondAirTemp\nj1939", "Aftrtratment2SecondAirDiffPress\nj1939", "Aftrtreatment2SecondAirMassFlow\nj1939"]}, {"XNET Frame"="AAI\nj1939", "Signals"=["AuxLevel\nj1939", "AuxPress1\nj1939", "AuxPress2\nj1939", "AuxTemp1\nj1939", "AuxTemp2\nj1939"]}, {"XNET Frame"="AC\nj1939", "Signals"=["ArticulationAngle\nj1939"]}, {"XNET Frame"="ACC1\nj1939", "Signals"=["ACCDistanceAlertSignal\nj1939", "ACCSystemShutoffWarning\nj1939", "ACCTargetDetected\nj1939", "AdaptiveCruiseCtrlMode\nj1939", "AdaptiveCruiseCtrlSetSpeed\nj1939", "AdptveCruiseCtrlSetDistanceMode\nj1939", "DistanceToForwardVehicle\nj1939", "ACC1.RoadCurvature\nj1939", "SpeedOfForwardVehicle\nj1939"]}, {"XNET Frame"="ACC2\nj1939", "Signals"=["RqedACCDistanceMode\nj1939"]}, {"XNET Frame"="ACKM\nj1939", "Signals"=["AddressAccessDenied\nj1939", "AddressAcknowledged\nj1939", "AddressBusy\nj1939", "AddressNegativeAcknowledgement\nj1939", "ACKM.ControlByte\nj1939", "GroupFunctionValue\nj1939", "ACKM.ParameterGroupNumber\nj1939"]}, {"XNET Frame"="ACL\nj1939", "Signals"=["ACL.ArbitraryAddressCapable\nj1939", "ACL.ECUInstance\nj1939", "ACL.Function\nj1939", "ACL.FunctionInstance\nj1939", "ACL.IdentityNumber\nj1939", "ACL.IndustryGroup\nj1939", "ACL.ManufacturerCode\nj1939", "ACL.VehicleSystem\nj1939", "ACL.VehicleSystemInstance\nj1939"]}, {"XNET Frame"="AETC\nj1939", "Signals"=["AETCDataCollectionStandard\nj1939", "NumberOfAETCDataPoints\nj1939"]}, {"XNET Frame"="AF2\nj1939", "Signals"=["EngDsiredAbsIntakeManifoldPress\nj1939", "EngGasFuelCorrectionFactor\nj1939", "EngGsMssFlwSnsrFelingCorrection\nj1939", "EngTurboWastegateValvePos\nj1939"]}, {"XNET Frame"="AFC1\nj1939", "Signals"=["Aftertreatment1FuelPress\nj1939", "Aftertreatment1FuelPressCtrl\nj1939", "Aftertreatment1FuelRate\nj1939", "Aftertreatment1Ignt\nj1939", "Aftrtratment1FuelEnableActuator\nj1939", "Aftrtratment1RegenerationStatus\nj1939"]}, {"XNET Frame"="AFC2\nj1939", "Signals"=["Aftertreatment2FuelPress\nj1939", "Aftertreatment2FuelPressCtrl\nj1939", "Aftertreatment2FuelRate\nj1939", "Aftertreatment2Ignt\nj1939", "Aftrtratment2FuelEnableActuator\nj1939", "Aftrtratment2RegenerationStatus\nj1939"]}, {"XNET Frame"="AFSS\nj1939", "Signals"=["LeftHeadlampDynamicBendingLight\nj1939", "LeftHeadlampLightDistribution\nj1939", "RghtHeadlampDynamicBendingLight\nj1939", "RightHeadlampLightDistribution\nj1939"]}, {"XNET Frame"="AI\nj1939", "Signals"=["DriveAxleLiftAirPress\nj1939", "DriveAxleLocation\nj1939", "DriveAxleLubePress\nj1939", "DriveAxleTemp\nj1939", "SteerAxleLubePress\nj1939", "SteerAxleTemp\nj1939"]}, {"XNET Frame"="AIR1\nj1939", "Signals"=["AirCompressorStatus\nj1939", "AirSuspensionSupplyPress\nj1939", "AuxEquipmentSupplyPress\nj1939", "ParkingAnd_OrTrailerAirPress\nj1939", "PneumaticSupplyPress\nj1939", "ServiceBrakeAirPressCircuit1\nj1939", "ServiceBrakeAirPressCircuit2\nj1939"]}, {"XNET Frame"="AIR2\nj1939", "Signals"=["EngAirStartPress\nj1939"]}, {"XNET Frame"="AMB\nj1939", "Signals"=["AmbientAirTemp\nj1939", "BarometricPress\nj1939", "CabInteriorTemp\nj1939", "EngAirInletTemp\nj1939", "RoadSurfaceTemp\nj1939"]}, {"XNET Frame"="AMB2\nj1939", "Signals"=["SolarIntensityPercent\nj1939", "SolarSensorMax\nj1939"]}, {"XNET Frame"="AP\nj1939", "Signals"=["AuxAbsPressReading\nj1939", "AuxGagePressReading1\nj1939", "AuxVacuumPressReading\nj1939"]}, {"XNET Frame"="AS\nj1939", "Signals"=["Alt1Status\nj1939", "Alt2Status\nj1939", "Alt3Status\nj1939", "Alt4Status\nj1939", "AltSpeed\nj1939"]}, {"XNET Frame"="ASC1\nj1939", "Signals"=["AboveNominalLevelFrontAxle\nj1939", "AboveNominalLevelRearAxle\nj1939", "BelowNominalLevelFrontAxle\nj1939", "BelowNominalLevelRearAxle\nj1939", "DoorRelease\nj1939", "FrontAxleInBumperRange\nj1939", "KneelingInformation\nj1939", "LevelCtrlMode\nj1939", "ASC1.LiftAxle1Pos\nj1939", "ASC1.LiftAxle2Pos\nj1939", "LiftingCtrlModeFrontAxle\nj1939", "LiftingCtrlModeRearAxle\nj1939", "LoweringCtrlModeFrontAxle\nj1939", "LoweringCtrlModeRearAxle\nj1939", "NominalLevelFrontAxle\nj1939", "NominalLevelRearAxle\nj1939", "RearAxleInBumperRange\nj1939", "SecurityDevice\nj1939", "SspensionCtrlRefusalInformation\nj1939", "SuspensionRemoteCtrl1\nj1939", "SuspensionRemoteCtrl2\nj1939", "VehicleMotionInhibit\nj1939"]}, {"XNET Frame"="ASC2\nj1939", "Signals"=["AutomaticTractionHelp\nj1939", "DamperStiffnessRqFrontAxle\nj1939", "DamperStiffnessRqLift_TagAxle\nj1939", "DamperStiffnessRqRearAxle\nj1939", "KneelingCmdFrontAxle\nj1939", "KneelingCmdRearAxle\nj1939", "KneelingCtrlModeRq\nj1939", "KneelingRqLeftSide\nj1939", "KneelingRqRightSide\nj1939", "LevelCtrlModeRq\nj1939", "LiftAxle1PosCmd\nj1939", "LiftAxle2PosCmd\nj1939", "NominalLevelRqFrontAxle\nj1939", "NominalLevelRqRearAxle\nj1939", "ProhibitAirSuspensionCtrl\nj1939"]}, {"XNET Frame"="ASC3\nj1939", "Signals"=["RelativeLevelFrontAxleLeft\nj1939", "RelativeLevelFrontAxleRight\nj1939", "RelativeLevelRearAxleLeft\nj1939", "RelativeLevelRearAxleRight\nj1939"]}, {"XNET Frame"="ASC4\nj1939", "Signals"=["BellowPressFrontAxleLeft\nj1939", "BellowPressFrontAxleRight\nj1939", "BellowPressRearAxleLeft\nj1939", "BellowPressRearAxleRight\nj1939"]}, {"XNET Frame"="ASC5\nj1939", "Signals"=["DamperStiffnessFrontAxle\nj1939", "DamperStiffnessLift_TagAxle\nj1939", "DamperStiffnessRearAxle\nj1939", "ElctrncShckAbsrbrCtrlMdFrntAxle\nj1939", "ElctrncShckAbsrbrCtrlMdLft_TgAxl\nj1939", "ElctrncShckAbsrbrCtrlMdRearAxle\nj1939"]}, {"XNET Frame"="ASC6\nj1939", "Signals"=["LevelPresetFrontAxleLeft\nj1939", "LevelPresetFrontAxleRight\nj1939", "LevelPresetRearAxleLeft\nj1939", "LevelPresetRearAxleRight\nj1939"]}, {"XNET Frame"="AT\nj1939", "Signals"=["EngAltBearing1Temp\nj1939", "EngAltBearing2Temp\nj1939", "EngAltWinding1Temp\nj1939", "EngAltWinding2Temp\nj1939", "EngAltWinding3Temp\nj1939"]}, {"XNET Frame"="AT1I1\nj1939", "Signals"=["Aftertreatment1IntakeNOx\nj1939", "Aftertreatment1IntakeO2\nj1939", "Aftrtrtmnt1IntkGsSnsrHeaterCtrl\nj1939", "Aftrtrtmnt1IntkGsSnsrHtrPrlmnryF\nj1939", "Aftrtrtmnt1IntkGsSnsrPwrInRange\nj1939", "Aftrtrtmnt1IntkNOxReadingStable\nj1939", "Aftrtrtmnt1IntkNOxSnsrPrlmnryFMI\nj1939", "Aftrtrtmnt1IntkOxygnSnsrPrlmnryF\nj1939", "Aftrtrtmnt1IntkWdRngO2RdngStble\nj1939", "Aftrtrtmnt1IntkeGasSensorAtTemp\nj1939"]}, {"XNET Frame"="AT1I2\nj1939", "Signals"=["Aftertreatment1ExhaustGasTemp1\nj1939", "Aftrtrtmnt1ExhstGsTmp1PrlmnryFMI\nj1939", "Aftrtrtmnt1PrtcltTrpIntkGasTemp\nj1939", "Aftrtrtmnt1PrtcltTrpIntkGsTmpPrl\nj1939"]}, {"XNET Frame"="AT1O1\nj1939", "Signals"=["Aftertreatment1OutletNOx\nj1939", "Aftertreatment1OutletO2\nj1939", "Aftrtrtmnt1OtletGasSensorAtTemp\nj1939", "Aftrtrtmnt1OtltGsSnsrHeaterCtrl\nj1939", "Aftrtrtmnt1OtltGsSnsrHtrPrlmnryF\nj1939", "Aftrtrtmnt1OtltGsSnsrPwrInRange\nj1939", "Aftrtrtmnt1OtltNOxReadingStable\nj1939", "Aftrtrtmnt1OtltNOxSnsrPrlmnryFMI\nj1939", "Aftrtrtmnt1OtltOxygnSnsrPrlmnryF\nj1939", "Aftrtrtmnt1OtltWdRngO2RdngStble\nj1939"]}, {"XNET Frame"="AT1O2\nj1939", "Signals"=["Aftertreatment1ExhaustGasTemp3\nj1939", "Aftrtrtmnt1ExhstGsTmp3PrlmnryFMI\nj1939", "Aftrtrtmnt1PrtcltTrpOtltExhstGsT\nj1939", "Aftrtrtmnt1PrtcltTrpOtltGasTemp\nj1939"]}, {"XNET Frame"="AT2I1\nj1939", "Signals"=["Aftertreatment2IntakeNOx\nj1939", "Aftertreatment2IntakeO2\nj1939", "Aftrtrtmnt2IntkGsSnsrHeaterCtrl\nj1939", "Aftrtrtmnt2IntkGsSnsrHtrPrlmnryF\nj1939", "Aftrtrtmnt2IntkGsSnsrPwrInRange\nj1939", "Aftrtrtmnt2IntkNOxReadingStable\nj1939", "Aftrtrtmnt2IntkNOxSnsrPrlmnryFMI\nj1939", "Aftrtrtmnt2IntkOxygnSnsrPrlmnryF\nj1939", "Aftrtrtmnt2IntkWdRngO2RdngStble\nj1939", "Aftrtrtmnt2IntkeGasSensorAtTemp\nj1939"]}, {"XNET Frame"="AT2I2\nj1939", "Signals"=["Aftertreatment2ExhaustGasTemp1\nj1939", "Aftrtrtmnt2ExhstGsTmp1PrlmnryFMI\nj1939", "Aftrtrtmnt2PrtcltTrpIntkGasTemp\nj1939", "Aftrtrtmnt2PrtcltTrpIntkGsTmpPrl\nj1939"]}, {"XNET Frame"="AT2O1\nj1939", "Signals"=["Aftertreatment2OutletNOx\nj1939", "Aftertreatment2OutletO2\nj1939", "Aftrtrtmnt2OtletGasSensorAtTemp\nj1939", "Aftrtrtmnt2OtltGsSnsrHeaterCtrl\nj1939", "Aftrtrtmnt2OtltGsSnsrHtrPrlmnryF\nj1939", "Aftrtrtmnt2OtltGsSnsrPwrInRange\nj1939", "Aftrtrtmnt2OtltNOxReadingStable\nj1939", "Aftrtrtmnt2OtltNOxSnsrPrlmnryFMI\nj1939", "Aftrtrtmnt2OtltOxygnSnsrPrlmnryF\nj1939", "Aftrtrtmnt2OtltWdRngO2RdngStble\nj1939"]}, {"XNET Frame"="AT2O2\nj1939", "Signals"=["Aftertreatment2ExhaustGasTemp3\nj1939", "Aftrtrtmnt2ExhstGsTmp3PrlmnryFMI\nj1939", "Aftrtrtmnt2PrtcltTrpExhstGsTmpPr\nj1939", "Aftrtrtmnt2PrtcltTrpOtltGasTemp\nj1939"]}, {"XNET Frame"="ATGP1\nj1939", "Signals"=["ParticulateTrapIntakePress1\nj1939", "ParticulateTrapOutletPress1\nj1939"]}, {"XNET Frame"="ATGP2\nj1939", "Signals"=["ParticulateTrapIntakePress2\nj1939", "ParticulateTrapOutletPress2\nj1939"]}, {"XNET Frame"="ATM1\nj1939", "Signals"=["ExhaustGasTemp2\nj1939", "ExhaustGasTemp2PreliminaryFMI\nj1939", "ParticulateTrapDiffPress\nj1939", "PrtclateTrapIntermediateGasTemp\nj1939", "PrtcltTrpDltPressPreliminaryFMI\nj1939", "PrtcltTrpIntrmdtGsTmpPrlmnryFMI\nj1939"]}, {"XNET Frame"="ATM2\nj1939", "Signals"=["Aftertreatment2ExhaustGasTemp2\nj1939", "Aftrtrtmnt2ExhstGsTmp2PrlmnryFMI\nj1939", "Aftrtrtmnt2PrtcltTrpDltPrssPrlmn\nj1939", "Aftrtrtmnt2PrtcltTrpIntrmdtGsTmp\nj1939", "Aftrtrtmnt2PrtclteTrapDiffPress\nj1939"]}, {"XNET Frame"="ATR\nj1939", "Signals"=["AntitheftCmdStates\nj1939", "AntitheftDesiredExitModeStates\nj1939", "AntitheftPasswordRepresentation\nj1939", "AntthftEncryptonIndicatorStates\nj1939"]}, {"XNET Frame"="ATS\nj1939", "Signals"=["AntitheftComponentStatusStates\nj1939", "AntitheftModifyPwdStates\nj1939", "AntitheftPwdValidIndicator\nj1939", "AntitheftRandomNumber\nj1939", "AntthftEncryptnSdPrsntIndicator\nj1939"]}, {"XNET Frame"="ATS1\nj1939", "Signals"=["ParticulateTrap1AshLoadPercent\nj1939", "ParticulateTrap1SootLoadPercent\nj1939", "PrtcltTrp1TmSncLstActvRgnration\nj1939"]}, {"XNET Frame"="ATS2\nj1939", "Signals"=["ParticulateTrap2AshLoadPercent\nj1939", "ParticulateTrap2SootLoadPercent\nj1939", "PrtcltTrp2TmSncLstActvRgnration\nj1939"]}, {"XNET Frame"="AUXIO1\nj1939", "Signals"=["AuxI_OChannel1\nj1939", "AuxI_OChannel2\nj1939"]}, {"XNET Frame"="AUXIO2\nj1939", "Signals"=["AuxI_O17\nj1939", "AuxI_O18\nj1939", "AuxI_O19\nj1939", "AuxI_O20\nj1939", "AuxI_O21\nj1939", "AuxI_O22\nj1939", "AuxI_O23\nj1939", "AuxI_O24\nj1939", "AuxI_O25\nj1939", "AuxI_O26\nj1939", "AuxI_O27\nj1939", "AuxI_O28\nj1939", "AuxI_O29\nj1939", "AuxI_O30\nj1939", "AuxI_O31\nj1939", "AuxI_O32\nj1939", "AuxI_O33\nj1939", "AuxI_O34\nj1939", "AuxI_O35\nj1939", "AuxI_O36\nj1939", "AuxI_O37\nj1939", "AuxI_O38\nj1939", "AuxI_O39\nj1939", "AuxI_O40\nj1939", "AuxI_O41\nj1939", "AuxI_O42\nj1939", "AuxI_O43\nj1939", "AuxI_O44\nj1939", "AuxI_O45\nj1939", "AuxI_O46\nj1939", "AuxI_O47\nj1939", "AuxI_O48\nj1939"]}, {"XNET Frame"="AUXIO3\nj1939", "Signals"=["AuxI_O49\nj1939", "AuxI_O50\nj1939", "AuxI_O51\nj1939", "AuxI_O52\nj1939", "AuxI_O53\nj1939", "AuxI_O54\nj1939", "AuxI_O55\nj1939", "AuxI_O56\nj1939", "AuxI_O57\nj1939", "AuxI_O58\nj1939", "AuxI_O59\nj1939", "AuxI_O60\nj1939", "AuxI_O61\nj1939", "AuxI_O62\nj1939", "AuxI_O63\nj1939", "AuxI_O64\nj1939", "AuxI_O65\nj1939", "AuxI_O66\nj1939", "AuxI_O67\nj1939", "AuxI_O68\nj1939", "AuxI_O69\nj1939", "AuxI_O70\nj1939", "AuxI_O71\nj1939", "AuxI_O72\nj1939", "AuxI_O73\nj1939", "AuxI_O74\nj1939", "AuxI_O75\nj1939", "AuxI_O76\nj1939", "AuxI_O77\nj1939", "AuxI_O78\nj1939", "AuxI_O79\nj1939", "AuxI_O80\nj1939"]}, {"XNET Frame"="AUXIO4\nj1939", "Signals"=["AuxI_O100\nj1939", "AuxI_O101\nj1939", "AuxI_O102\nj1939", "AuxI_O103\nj1939", "AuxI_O104\nj1939", "AuxI_O105\nj1939", "AuxI_O106\nj1939", "AuxI_O107\nj1939", "AuxI_O108\nj1939", "AuxI_O109\nj1939", "AuxI_O110\nj1939", "AuxI_O111\nj1939", "AuxI_O112\nj1939", "AuxI_O81\nj1939", "AuxI_O82\nj1939", "AuxI_O83\nj1939", "AuxI_O84\nj1939", "AuxI_O85\nj1939", "AuxI_O86\nj1939", "AuxI_O87\nj1939", "AuxI_O88\nj1939", "AuxI_O89\nj1939", "AuxI_O90\nj1939", "AuxI_O91\nj1939", "AuxI_O92\nj1939", "AuxI_O93\nj1939", "AuxI_O94\nj1939", "AuxI_O95\nj1939", "AuxI_O96\nj1939", "AuxI_O97\nj1939", "AuxI_O98\nj1939", "AuxI_O99\nj1939"]}, {"XNET Frame"="AWPP\nj1939", "Signals"=["AuxPumpPress\nj1939"]}, {"XNET Frame"="B\nj1939", "Signals"=["BrakeAppPress\nj1939", "BrakePrimaryPress\nj1939", "BrakeSecondPress\nj1939", "ParkBrakeReleaseInhibitStatus\nj1939", "ParkingBrakeActuator\nj1939", "ParkingBrakeRedWarningSignal\nj1939"]}, {"XNET Frame"="BAAC\nj1939", "Signals"=["Bs1AvrgeLineNeutralACRMSVoltage\nj1939", "Bus1AverageACFrequency\nj1939", "Bus1AverageLineLineACRMSVoltage\nj1939"]}, {"XNET Frame"="BGSC\nj1939", "Signals"=["Bus1_GeneratorACPhaseDifference\nj1939", "Bus1_GeneratorDeadBus\nj1939", "Bus1_GeneratorFrequencyMatch\nj1939", "Bus1_GeneratorInSync\nj1939", "Bus1_GeneratorPhaseMatch\nj1939", "Bus1_GeneratorVoltageMatch\nj1939"]}, {"XNET Frame"="BI\nj1939", "Signals"=["BladeRotationAngle\nj1939", "BladeRotationAngleFigureOfMerit\nj1939", "RelBladeHeightFigureOfMerit\nj1939", "RelBladeMeasurementLatency\nj1939", "RelativeBladeHeight\nj1939"]}, {"XNET Frame"="BJM1\nj1939", "Signals"=["Joystick1Button10PressedStatus\nj1939", "Joystick1Button11PressedStatus\nj1939", "Joystick1Button12PressedStatus\nj1939", "Joystick1Button1PressedStatus\nj1939", "Joystick1Button2PressedStatus\nj1939", "Joystick1Button3PressedStatus\nj1939", "Joystick1Button4PressedStatus\nj1939", "Joystick1Button5PressedStatus\nj1939", "Joystick1Button6PressedStatus\nj1939", "Joystick1Button7PressedStatus\nj1939", "Joystick1Button8PressedStatus\nj1939", "Joystick1Button9PressedStatus\nj1939", "Joystick1XAxisDetentPosStatus\nj1939", "Joystick1XAxisNeutralPosStatus\nj1939", "Joystick1XAxisPos\nj1939", "Joystick1YAxisDetentPosStatus\nj1939", "Joystick1YAxisNeutralPosStatus\nj1939", "Joystick1YAxisPos\nj1939", "Jystck1XAxsLvrLftNgtvePosStatus\nj1939", "Jystck1XAxsLvrRghtPstvPosStatus\nj1939", "Jystck1YAxsLvrBckNgtvePosStatus\nj1939", "Jystck1YAxsLvrFrwrdPstvPsStatus\nj1939"]}, {"XNET Frame"="BJM2\nj1939", "Signals"=["Joystick2Button10PressedStatus\nj1939", "Joystick2Button11PressedStatus\nj1939", "Joystick2Button12PressedStatus\nj1939", "Joystick2Button1PressedStatus\nj1939", "Joystick2Button2PressedStatus\nj1939", "Joystick2Button3PressedStatus\nj1939", "Joystick2Button4PressedStatus\nj1939", "Joystick2Button5PressedStatus\nj1939", "Joystick2Button6PressedStatus\nj1939", "Joystick2Button7PressedStatus\nj1939", "Joystick2Button8PressedStatus\nj1939", "Joystick2Button9PressedStatus\nj1939", "Joystick2XAxisDetentPosStatus\nj1939", "Joystick2XAxisNeutralPosStatus\nj1939", "Joystick2XAxisPos\nj1939", "Joystick2YAxisDetentPosStatus\nj1939", "Joystick2YAxisNeutralPosStatus\nj1939", "Joystick2YAxisPos\nj1939", "Jystck2XAxsLvrLftNgtvePosStatus\nj1939", "Jystck2XAxsLvrRghtPstvPosStatus\nj1939", "Jystck2YAxsLvrBckNgtvePosStatus\nj1939", "Jystck2YAxsLvrFrwrdPstvPsStatus\nj1939"]}, {"XNET Frame"="BJM3\nj1939", "Signals"=["Joystick3Button10PressedStatus\nj1939", "Joystick3Button11PressedStatus\nj1939", "Joystick3Button12PressedStatus\nj1939", "Joystick3Button1PressedStatus\nj1939", "Joystick3Button2PressedStatus\nj1939", "Joystick3Button3PressedStatus\nj1939", "Joystick3Button4PressedStatus\nj1939", "Joystick3Button5PressedStatus\nj1939", "Joystick3Button6PressedStatus\nj1939", "Joystick3Button7PressedStatus\nj1939", "Joystick3Button8PressedStatus\nj1939", "Joystick3Button9PressedStatus\nj1939", "Joystick3XAxisDetentPosStatus\nj1939", "Joystick3XAxisNeutralPosStatus\nj1939", "Joystick3XAxisPos\nj1939", "Joystick3YAxisDetentPosStatus\nj1939", "Joystick3YAxisNeutralPosStatus\nj1939", "Joystick3YAxisPos\nj1939", "Jystck3XAxsLvrLftNgtvePosStatus\nj1939", "Jystck3XAxsLvrRghtPstvPosStatus\nj1939", "Jystck3YAxsLvrBckNgtvePosStatus\nj1939", "Jystck3YAxsLvrFrwrdPstvPsStatus\nj1939"]}, {"XNET Frame"="BM\nj1939", "Signals"=["BatteryMainSwitchHoldState\nj1939"]}, {"XNET Frame"="BPAAC\nj1939", "Signals"=["Bs1PhseALineNeutralACRMSVoltage\nj1939", "Bus1PhaseAACFrequency\nj1939", "Bus1PhaseABLineLineACRMSVoltage\nj1939"]}, {"XNET Frame"="BPBAC\nj1939", "Signals"=["Bs1PhseBLineNeutralACRMSVoltage\nj1939", "Bus1PhaseBACFrequency\nj1939", "Bus1PhaseBCLineLineACRMSVoltage\nj1939"]}, {"XNET Frame"="BPCAC\nj1939", "Signals"=["Bs1PhseCLineNeutralACRMSVoltage\nj1939", "Bus1PhaseCACFrequency\nj1939", "Bus1PhaseCALineLineACRMSVoltage\nj1939"]}, {"XNET Frame"="BSA\nj1939", "Signals"=["TractorBrakeStrokeAxle1Left\nj1939", "TractorBrakeStrokeAxle1Right\nj1939", "TractorBrakeStrokeAxle2Left\nj1939", "TractorBrakeStrokeAxle2Right\nj1939", "TractorBrakeStrokeAxle3Left\nj1939", "TractorBrakeStrokeAxle3Right\nj1939", "TractorBrakeStrokeAxle4Left\nj1939", "TractorBrakeStrokeAxle4Right\nj1939", "TractorBrakeStrokeAxle5Left\nj1939", "TractorBrakeStrokeAxle5Right\nj1939", "TrailerBrakeStrokeAxle1Left\nj1939", "TrailerBrakeStrokeAxle1Right\nj1939", "TrailerBrakeStrokeAxle2Left\nj1939", "TrailerBrakeStrokeAxle2Right\nj1939", "TrailerBrakeStrokeAxle3Left\nj1939", "TrailerBrakeStrokeAxle3Right\nj1939", "TrailerBrakeStrokeAxle4Left\nj1939", "TrailerBrakeStrokeAxle4Right\nj1939", "TrailerBrakeStrokeAxle5Left\nj1939", "TrailerBrakeStrokeAxle5Right\nj1939"]}, {"XNET Frame"="BT1\nj1939", "Signals"=["Battery1Temp\nj1939", "Battery2Temp\nj1939"]}, {"XNET Frame"="BUSC\nj1939", "Signals"=["Bus1_UtilityACPhaseDifference\nj1939", "Bus1_UtilityDeadBus\nj1939", "Bus1_UtilityFrequencyMatch\nj1939", "Bus1_UtilityInSync\nj1939", "Bus1_UtilityPhaseMatch\nj1939", "Bus1_UtilityVoltageMatch\nj1939"]}, {"XNET Frame"="CACI\nj1939", "Signals"=["CbA_CRfrgrntCmprssorOutletPress\nj1939"]}, {"XNET Frame"="CCC\nj1939", "Signals"=["AuxHeaterMaxOutputPower\nj1939"]}, {"XNET Frame"="CCS\nj1939", "Signals"=["EngCyl10CombustionStatus\nj1939", "EngCyl11CombustionStatus\nj1939", "EngCyl12CombustionStatus\nj1939", "EngCyl13CombustionStatus\nj1939", "EngCyl14CombustionStatus\nj1939", "EngCyl15CombustionStatus\nj1939", "EngCyl16CombustionStatus\nj1939", "EngCyl17CombustionStatus\nj1939", "EngCyl18CombustionStatus\nj1939", "EngCyl19CombustionStatus\nj1939", "EngCyl1CombustionStatus\nj1939", "EngCyl20CombustionStatus\nj1939", "EngCyl21CombustionStatus\nj1939", "EngCyl22CombustionStatus\nj1939", "EngCyl23CombustionStatus\nj1939", "EngCyl24CombustionStatus\nj1939", "EngCyl2CombustionStatus\nj1939", "EngCyl3CombustionStatus\nj1939", "EngCyl4CombustionStatus\nj1939", "EngCyl5CombustionStatus\nj1939", "EngCyl6CombustionStatus\nj1939", "EngCyl7CombustionStatus\nj1939", "EngCyl8CombustionStatus\nj1939", "EngCyl9CombustionStatus\nj1939"]}, {"XNET Frame"="CCSS\nj1939", "Signals"=["CruiseCtrlHighSetLimitSpeed\nj1939", "CruiseCtrlLowSetLimitSpeed\nj1939", "CCSS.MaxVehicleSpeedLimit\nj1939"]}, {"XNET Frame"="CCVS\nj1939", "Signals"=["BrakeSwitch\nj1939", "ClutchSwitch\nj1939", "CruiseCtrlAccelerateSwitch\nj1939", "CruiseCtrlActive\nj1939", "CruiseCtrlCoastSwitch\nj1939", "CruiseCtrlEnableSwitch\nj1939", "CruiseCtrlPauseSwitch\nj1939", "CruiseCtrlResumeSwitch\nj1939", "CruiseCtrlSetSpeed\nj1939", "CruiseCtrlSetSwitch\nj1939", "CruiseCtrlStates\nj1939", "EngIdleDecrementSwitch\nj1939", "EngIdleIncrementSwitch\nj1939", "EngShutdownOverrideSwitch\nj1939", "EngTestModeSwitch\nj1939", "PTOState\nj1939", "ParkBrakeReleaseInhibitRq\nj1939", "ParkingBrakeSwitch\nj1939", "TwoSpeedAxleSwitch\nj1939", "CCVS.WheelBasedVehicleSpeed\nj1939"]}, {"XNET Frame"="CL\nj1939", "Signals"=["IlluminationBrightnessPercent\nj1939"]}, {"XNET Frame"="CM1\nj1939", "Signals"=["AtmaticGearShiftingEnableSwitch\nj1939", "AuxHeaterCoolantPumpRq\nj1939", "AuxHeaterModeRq\nj1939", "BatteryMainSwitchHoldRq\nj1939", "CabInteriorTempCmd\nj1939", "EngAutomaticStartEnableSwitch\nj1939", "OperatorSeatDirectionSwitch\nj1939", "RqCabZoneHeating\nj1939", "RqEngZoneHeating\nj1939", "RqedPercentFanSpeed\nj1939", "SeatBeltSwitch\nj1939", "SelectedMaxVehicleSpeedLimit\nj1939", "VhclLmtngSpdGvernorEnableSwitch\nj1939", "VhclLmtngSpdGvrnrDcrementSwitch\nj1939", "VhclLmtngSpdGvrnrIncrmentSwitch\nj1939"]}, {"XNET Frame"="CM3\nj1939", "Signals"=["FfthWhlRlaseCtrlSecurityLockout\nj1939", "FifthWheelReleaseCtrl\nj1939", "TransOilLevelRq\nj1939", "TransferCaseSelectorSwitch\nj1939"]}, {"XNET Frame"="CMI\nj1939", "Signals"=["TotalCountOfConfigChangesMade\nj1939"]}, {"XNET Frame"="CRI1\nj1939", "Signals"=["CatalystReagentConcentration\nj1939", "CatalystReagentConductivity\nj1939", "CatalystReagentTemp2\nj1939", "CatalystReagentType\nj1939", "CtlystRagentTemp2PreliminaryFMI\nj1939", "CtlystRgntPrprtesPreliminaryFMI\nj1939"]}, {"XNET Frame"="CSA\nj1939", "Signals"=["EngStartEnableDevice1\nj1939", "EngStartEnableDevice1Config\nj1939", "EngStartEnableDevice2\nj1939", "EngStartEnableDevice2Config\nj1939"]}, {"XNET Frame"="CT1\nj1939", "Signals"=["EngCyl1CombustionTime\nj1939", "EngCyl2CombustionTime\nj1939", "EngCyl3CombustionTime\nj1939", "EngCyl4CombustionTime\nj1939"]}, {"XNET Frame"="CT2\nj1939", "Signals"=["EngCyl5CombustionTime\nj1939", "EngCyl6CombustionTime\nj1939", "EngCyl7CombustionTime\nj1939", "EngCyl8CombustionTime\nj1939"]}, {"XNET Frame"="CT3\nj1939", "Signals"=["EngCyl10CombustionTime\nj1939", "EngCyl11CombustionTime\nj1939", "EngCyl12CombustionTime\nj1939", "EngCyl9CombustionTime\nj1939"]}, {"XNET Frame"="CT4\nj1939", "Signals"=["EngCyl13CombustionTime\nj1939", "EngCyl14CombustionTime\nj1939", "EngCyl15CombustionTime\nj1939", "EngCyl16CombustionTime\nj1939"]}, {"XNET Frame"="CT5\nj1939", "Signals"=["EngCyl17CombustionTime\nj1939", "EngCyl18CombustionTime\nj1939", "EngCyl19CombustionTime\nj1939", "EngCyl20CombustionTime\nj1939"]}, {"XNET Frame"="CT6\nj1939", "Signals"=["EngAverageCombustionTime\nj1939", "EngDesiredCombustionTime\nj1939"]}, {"XNET Frame"="CTL\nj1939", "Signals"=["EngSpeedLimitRqMaxContinuous\nj1939", "EngSpeedLimitRqMinContinuous\nj1939", "EngTorqueLimitRqMaxContinuous\nj1939", "EngTorqueLimitRqMinContinuous\nj1939", "MnCntinuousRetarderSpeedLimitRq\nj1939", "MnCntnuousRetarderTorqueLimitRq\nj1939", "MxCntinuousRetarderSpeedLimitRq\nj1939", "MxCntnuousRetarderTorqueLimitRq\nj1939"]}, {"XNET Frame"="CVW\nj1939", "Signals"=["GrossCombinationVehicleWeight\nj1939", "PoweredVehicleWeight\nj1939"]}, {"XNET Frame"="DC1\nj1939", "Signals"=["PosOfDoors\nj1939", "Ramp_WheelChairLiftPos\nj1939", "Status2OfDoors\nj1939"]}, {"XNET Frame"="DC2\nj1939", "Signals"=["EnableStatusOfDoor1\nj1939", "EnableStatusOfDoor10\nj1939", "EnableStatusOfDoor2\nj1939", "EnableStatusOfDoor3\nj1939", "EnableStatusOfDoor4\nj1939", "EnableStatusOfDoor5\nj1939", "EnableStatusOfDoor6\nj1939", "EnableStatusOfDoor7\nj1939", "EnableStatusOfDoor8\nj1939", "EnableStatusOfDoor9\nj1939", "LockStatusOfDoor1\nj1939", "LockStatusOfDoor10\nj1939", "LockStatusOfDoor2\nj1939", "LockStatusOfDoor3\nj1939", "LockStatusOfDoor4\nj1939", "LockStatusOfDoor5\nj1939", "LockStatusOfDoor6\nj1939", "LockStatusOfDoor7\nj1939", "LockStatusOfDoor8\nj1939", "LockStatusOfDoor9\nj1939", "OpenStatusOfDoor1\nj1939", "OpenStatusOfDoor10\nj1939", "OpenStatusOfDoor2\nj1939", "OpenStatusOfDoor3\nj1939", "OpenStatusOfDoor4\nj1939", "OpenStatusOfDoor5\nj1939", "OpenStatusOfDoor6\nj1939", "OpenStatusOfDoor7\nj1939", "OpenStatusOfDoor8\nj1939", "OpenStatusOfDoor9\nj1939"]}, {"XNET Frame"="DD\nj1939", "Signals"=["CargoAmbientTemp\nj1939", "EngFuelFilterDiffPress\nj1939", "EngOilFilterDiffPress\nj1939", "FuelLevel\nj1939", "WasherFluidLevel\nj1939"]}, {"XNET Frame"="DISP1\nj1939", "Signals"=["TextDisplayIndex\nj1939", "TextDisplayInstructions\nj1939"]}, {"XNET Frame"="DM10\nj1939", "Signals"=["TestIdentifierSupported\nj1939"]}, {"XNET Frame"="DM13\nj1939", "Signals"=["CurrentDataLink\nj1939", "HoldSignal\nj1939", "ISO9141\nj1939", "J1939Network1\nj1939", "J1939Network2\nj1939", "J1939Network3\nj1939", "ManufacturerSpecificPort\nj1939", "SAE_J1587\nj1939", "SAE_J1850\nj1939", "SAE_J1922\nj1939", "SuspendDuration\nj1939", "SuspendSignal\nj1939"]}, {"XNET Frame"="DM14\nj1939", "Signals"=["Command\nj1939", "KeyOrUserLevel\nj1939", "NumberRequested\nj1939", "NumberRequestedHigh\nj1939", "Pointer\nj1939", "PointerExtension\nj1939", "PointerType\nj1939"]}, {"XNET Frame"="DM15\nj1939", "Signals"=["EDCP_Extension\nj1939", "ErrorIndicator\nj1939", "NumberAllowed\nj1939", "NumberAllowedHigh\nj1939", "Seed\nj1939", "Status\nj1939"]}, {"XNET Frame"="DM16\nj1939", "Signals"=["NumberOfOccurance\nj1939"]}, {"XNET Frame"="DM18\nj1939", "Signals"=["SecurityEntityLength\nj1939", "SecurityEntityLengthHigh\nj1939", "SecurityEntityType\nj1939"]}, {"XNET Frame"="DM21\nj1939", "Signals"=["DistanceSinceDTCsCleared\nj1939", "DistanceWhileMILisActivated\nj1939", "MinutesRunByEngineMILActivated\nj1939", "TimeSinceDTCsCleared\nj1939"]}, {"XNET Frame"="DM22\nj1939", "Signals"=["CtrlByteIndicIndividualDTCClear\nj1939", "DM22.FailureModeIdentifier1\nj1939", "IndividualDTCClearControlByte\nj1939", "DM22.SPN1\nj1939", "DM22.SPN1High\nj1939"]}, {"XNET Frame"="DM26\nj1939", "Signals"=["ACSystemRefrigerantMonComplete\nj1939", "ACSystemRefrigerantMonEnabled\nj1939", "CatalystMonComplete\nj1939", "CatalystMonEnabled\nj1939", "ColdStartAidSystemMonComplete\nj1939", "ColdStartAidSystemMonEnabled\nj1939", "ComprehensiveCompMonEnabled\nj1939", "ComprehensiveComptMonComplete\nj1939", "EGRSystemMonitoringComplete\nj1939", "EGRSystemMonitoringEnabled\nj1939", "EvaporativeSystemMonComplete\nj1939", "EvaporativeSystemMonEnabled\nj1939", "FuelSystemMonitoringComplete\nj1939", "FuelSystemMonitoringEnabled\nj1939", "HeatedCatalystMonComplete\nj1939", "HeatedCatalystMonEnabled\nj1939", "MisfireMonitoringComplete\nj1939", "MisfireMonitoringEnabled\nj1939", "NumOfWarmUpsSinceDTCsCleared\nj1939", "OxygenSensorHeaterMonComplete\nj1939", "OxygenSensorHeaterMonEnabled\nj1939", "OxygenSensorMonComplete\nj1939", "OxygenSensorMonEnabled\nj1939", "SecondAirSystemMonComplete\nj1939", "SecondAirSystemMonEnabled\nj1939", "TimeSinceEngineStart\nj1939"]}, {"XNET Frame"="DM29\nj1939", "Signals"=["AllPendingDTCs\nj1939", "MILOnDTCs\nj1939", "PendingDTCs\nj1939", "PermanentDTCs\nj1939", "PreviouslyMILOnDTCs\nj1939"]}, {"XNET Frame"="DM5\nj1939", "Signals"=["ACSystemRefrigerantMonStatus\nj1939", "ACSystemRefrigerantMonSupp\nj1939", "ActiveTroubleCodes\nj1939", "CatalystMonStatus\nj1939", "CatalystMonSupp\nj1939", "ColdStartAidSystemMonStatus\nj1939", "ColdStartAidSystemMonSupp\nj1939", "ComprehensiveCompMonStatus\nj1939", "ComprehensiveComponentMonSupp\nj1939", "EGRSystemMonitoringStatus\nj1939", "EGRSystemMonitoringSupp\nj1939", "EvaporativeSystemMonStatus\nj1939", "EvaporativeSystemMonSupp\nj1939", "FuelSystemMonitoringStatus\nj1939", "FuelSystemMonitoringSupport\nj1939", "HeatedCatalystMonStatus\nj1939", "HeatedCatalystMonSupp\nj1939", "MisfireMonitoringStatus\nj1939", "MisfireMonitoringSupport\nj1939", "OBDCompliance\nj1939", "OxygenSensorHeaterMonStatus\nj1939", "OxygenSensorHeaterMonSupp\nj1939", "OxygenSensorMonStatus\nj1939", "OxygenSensorMonSupp\nj1939", "PreviouslyActiveTroubleCodes\nj1939", "SecondAirSystemMonStatus\nj1939", "SecondAirSystemMonSupp\nj1939"]}, {"XNET Frame"="DM7\nj1939", "Signals"=["DM7.TestIdentifier\nj1939"]}, {"XNET Frame"="DM8\nj1939", "Signals"=["DM8.TestIdentifier\nj1939", "TestLimitMaximum\nj1939", "TestLimitMinimum\nj1939", "TestType\nj1939", "TestValue\nj1939"]}, {"XNET Frame"="DRC\nj1939", "Signals"=["EnableStatusOfRamp1\nj1939", "EnableStatusOfRamp2\nj1939", "EnableStatusOfRamp3\nj1939", "MovementStatusOfRamp1\nj1939", "MovementStatusOfRamp2\nj1939", "MovementStatusOfRamp3\nj1939", "RetractStatusOfRamp1\nj1939", "RetractStatusOfRamp2\nj1939", "RetractStatusOfRamp3\nj1939"]}, {"XNET Frame"="EAC\nj1939", "Signals"=["EngAuxCoolantPress\nj1939", "EngAuxCoolantTemp\nj1939", "SeaWaterPumpOutletPress\nj1939"]}, {"XNET Frame"="EAC1\nj1939", "Signals"=["DiffLockStateCentral\nj1939", "DiffLockStateCentralFront\nj1939", "DiffLockStateCentralRear\nj1939", "DiffLockStateFrontAxle1\nj1939", "DiffLockStateFrontAxle2\nj1939", "DiffLockStateRearAxle1\nj1939", "DiffLockStateRearAxle2\nj1939", "FrontAxleGroupEngagementStatus\nj1939", "Location\nj1939", "RearAxleGroupEngagementStatus\nj1939"]}, {"XNET Frame"="EBC1\nj1939", "Signals"=["ABSFullyOperational\nj1939", "ABSOffroadSwitch\nj1939", "ABS_EBSAmberWarningSignal\nj1939", "ASRBrakeCtrlActive\nj1939", "ASREngCtrlActive\nj1939", "ASRHillHolderSwitch\nj1939", "ASROffroadSwitch\nj1939", "ATC_ASRInformationSignal\nj1939", "AccelInterlockSwitch\nj1939", "AntiLockBrakingActive\nj1939", "BrakePedalPos\nj1939", "EBSBrakeSwitch\nj1939", "EBSRedWarningSignal\nj1939", "EngAuxEngShutdownSwitch\nj1939", "EngDerateSwitch\nj1939", "EngRetarderSelection\nj1939", "HaltBrakeSwitch\nj1939", "RemoteAccelEnableSwitch\nj1939", "SrcAddrssOfCtrllngDvcFrBrkCntrl\nj1939", "TractionCtrlOverrideSwitch\nj1939", "TrailerABSStatus\nj1939", "TrctrMntdTrilerABSWarningSignal\nj1939"]}, {"XNET Frame"="EBC2\nj1939", "Signals"=["FrontAxleSpeed\nj1939", "RelativeSpeedFrontAxleLeftWheel\nj1939", "RelativeSpeedRearAxle1LeftWheel\nj1939", "RelativeSpeedRearAxle2LeftWheel\nj1939", "RlativeSpeedFrontAxleRightWheel\nj1939", "RlativeSpeedRearAxle1RightWheel\nj1939", "RlativeSpeedRearAxle2RightWheel\nj1939"]}, {"XNET Frame"="EBC3\nj1939", "Signals"=["BrkAppPrssHghRngFrntAxlLftWheel\nj1939", "BrkAppPrssHghRngFrntAxlRghtWhel\nj1939", "BrkAppPrssHghRngRrAxl1LeftWheel\nj1939", "BrkAppPrssHghRngRrAxl1RghtWheel\nj1939", "BrkAppPrssHghRngRrAxl2LeftWheel\nj1939", "BrkAppPrssHghRngRrAxl2RghtWheel\nj1939", "BrkAppPrssHghRngRrAxl3LeftWheel\nj1939", "BrkAppPrssHghRngRrAxl3RghtWheel\nj1939"]}, {"XNET Frame"="EBC4\nj1939", "Signals"=["BrkLnngRmningFrontAxleLeftWheel\nj1939", "BrkLnngRmningRearAxle1LeftWheel\nj1939", "BrkLnngRmningRearAxle2LeftWheel\nj1939", "BrkLnngRmningRearAxle3LeftWheel\nj1939", "BrkLnngRmnngFrontAxleRightWheel\nj1939", "BrkLnngRmnngRearAxle1RightWheel\nj1939", "BrkLnngRmnngRearAxle2RightWheel\nj1939", "BrkLnngRmnngRearAxle3RightWheel\nj1939"]}, {"XNET Frame"="EBC5\nj1939", "Signals"=["BrakeTempWarning\nj1939", "FoundationBrakeUse\nj1939", "HaltBrakeMode\nj1939", "HillHolderMode\nj1939", "XBRAccelerationLimit\nj1939", "XBRActiveCtrlMode\nj1939", "XBRSystemState\nj1939"]}, {"XNET Frame"="EBS11\nj1939", "Signals"=["ASRBreakControlActive\nj1939", "ASREngineControlActive\nj1939", "BrakeLightSwitch\nj1939", "ParkBrakeDemandValue\nj1939", "RetarderDemandValue\nj1939", "ServiceBrakeDemandValue\nj1939", "EBS11.VehicleABSActive\nj1939", "EBS11.VehicleRetarderCtrlActive\nj1939", "EBS11.VehicleType\nj1939"]}, {"XNET Frame"="EBS12\nj1939", "Signals"=["ABSOffroadRequest\nj1939", "PneumaticControlLine\nj1939", "EBS12.RoadCurvature\nj1939", "TwoElCircuitsBrakeDemand\nj1939", "EBS12.VehicleRetarderCtrlActive\nj1939"]}, {"XNET Frame"="EBS21\nj1939", "Signals"=["ActualRetarderPercTorque\nj1939", "EBS21.AutomTowedVehBreakActive\nj1939", "EBS21.SupplyLineBrakingRequest\nj1939", "VDCActive\nj1939", "EBS21.VehicleABSActive\nj1939", "EBS21.VehicleRetarderCtrlActive\nj1939", "EBS21.VehicleServiceBrakeActive\nj1939", "WheelSpeedDiffMainAxle\nj1939", "Wheel_BasedVehicleSpeed\nj1939"]}, {"XNET Frame"="EBS22\nj1939", "Signals"=["AmberWarningSignalReq\nj1939", "EBS22.AutomTowedVehBreakActive\nj1939", "AxleLoadSum\nj1939", "ElecSupplyOfNonBrakingSys\nj1939", "ElectrLoadPropFunc\nj1939", "LoadingRampApproachAssist\nj1939", "RedWarningSignalRequest\nj1939", "EBS22.ReferenceRetarderTorque\nj1939", "SpringBrakeEngaged\nj1939", "SpringBrakeInstalled\nj1939", "EBS22.SupplyLineBrakingRequest\nj1939", "EBS22.VehicleABSActive\nj1939", "VehicleElectrSupplySuff\nj1939", "EBS22.VehicleRetarderCtrlActive\nj1939", "EBS22.VehicleServiceBrakeActive\nj1939", "EBS22.VehicleType\nj1939"]}, {"XNET Frame"="EBS23\nj1939", "Signals"=["BrakeLining\nj1939", "BrakeLiningSufficient\nj1939", "BrakeTemperature\nj1939", "BrakeTemperatureStatus\nj1939", "PneumaticSupplyPressure\nj1939", "TyrePressure\nj1939", "TyrePressureSufficient\nj1939", "TyreWheelIdentLining1\nj1939", "TyreWheelIdentLining2\nj1939", "TyreWheelIdentPressure1\nj1939", "TyreWheelIdentPressure2\nj1939", "TyreWheelIdentTemp1\nj1939", "TyreWheelIdentTemp2\nj1939", "VehiclePneumSupplySuff\nj1939"]}, {"XNET Frame"="EC2\nj1939", "Signals"=["MaxCrankAttemptsPerStartAttempt\nj1939"]}, {"XNET Frame"="ECT1\nj1939", "Signals"=["EngHghLmtThrshhldFrMnCntnsEngRPM\nj1939", "EngHghLmtThrshhldFrMnCntnsTrqFrm\nj1939", "EngLwLmtThrshhldFrMaxRPMFromEng\nj1939", "EngLwLmtThrshldFrMxTrqueFromEng\nj1939", "EngMaxContinuousRPM\nj1939", "EngMaxContinuousTorque\nj1939", "EngMinContinuousRPM\nj1939", "EngMinContinuousTorque\nj1939"]}, {"XNET Frame"="EEC1\nj1939", "Signals"=["ActualEngPercentTorque\nj1939", "DriversDemandEngPercentTorque\nj1939", "EngDemandPercentTorque\nj1939", "EEC1.EngSpeed\nj1939", "EngStarterMode\nj1939", "EEC1.EngTorqueMode\nj1939", "SrcAddrssOfCtrllngDvcForEngCtrl\nj1939"]}, {"XNET Frame"="EEC2\nj1939", "Signals"=["AccelPedal1LowIdleSwitch\nj1939", "AccelPedal2LowIdleSwitch\nj1939", "AccelPedalKickdownSwitch\nj1939", "AccelPedalPos1\nj1939", "AccelPedalPos2\nj1939", "ActMaxAvailEngPercentTorque\nj1939", "EEC2.EngPercentLoadAtCurrentSpeed\nj1939", "RemoteAccelPedalPos\nj1939", "RoadSpeedLimitStatus\nj1939", "VhclAccelerationRateLimitStatus\nj1939"]}, {"XNET Frame"="EEC3\nj1939", "Signals"=["AftrTrtmntExhustDewPointMessage\nj1939", "AftrTrtmntIntakeDewPointMessage\nj1939", "EngsDesiredOperatingSpeed\nj1939", "EngsDsrdOprtngSpdAsymmtryAdjstmn\nj1939", "EstEngPrsticLossesPercentTorque\nj1939", "ExhaustGasMass\nj1939", "NominalFrictionPercentTorque\nj1939"]}, {"XNET Frame"="EEC4\nj1939", "Signals"=["CrnkAttmptCntOnPrsntStrtAttempt\nj1939", "EngRatedPower\nj1939", "EngRatedSpeed\nj1939", "EngRotationDirection\nj1939"]}, {"XNET Frame"="EEC5\nj1939", "Signals"=["EngExhstGsRcirculationValveCtrl\nj1939", "EngTrb1ClclatedTurbineInletTemp\nj1939", "EngTrb1ClcltedTurbineOutletTemp\nj1939", "EngVrblGmtryTrbArCtrlShtffValve\nj1939", "EngVrblGometryTurbo1ActuatorPos\nj1939"]}, {"XNET Frame"="EEC6\nj1939", "Signals"=["EngTrbCmprssorBypassActuatorPos\nj1939", "EngTurboCompressorCtrl\nj1939", "EngVrableGeometryTurboActuator1\nj1939"]}, {"XNET Frame"="EEC7\nj1939", "Signals"=["EngExhstGsRcirculationValve2Pos\nj1939", "EngExhstGsRecirculationValvePos\nj1939"]}, {"XNET Frame"="EEC8\nj1939", "Signals"=["EngExhstGsRcrculationValve2Ctrl\nj1939"]}, {"XNET Frame"="EES\nj1939", "Signals"=["ElectricalLoad\nj1939", "SafetyWireStatus\nj1939", "TurningGearEngaged\nj1939"]}, {"XNET Frame"="EFL_P1\nj1939", "Signals"=["EngCoolantLevel\nj1939", "EngCoolantPress\nj1939", "EngCrankcasePress\nj1939", "EngExCrankcaseBlowbyPress\nj1939", "EngFuelDeliveryPress\nj1939", "EngOilLevel\nj1939", "EngOilPress\nj1939"]}, {"XNET Frame"="EFL_P2\nj1939", "Signals"=["EngInjectionCtrlPress\nj1939", "EngInjectorMeteringRail1Press\nj1939", "EngInjectorMeteringRail2Press\nj1939", "EngInjectorTimingRail1Press\nj1939"]}, {"XNET Frame"="EFL_P3\nj1939", "Signals"=["EngExhstGsRcrculationInletPress\nj1939", "EngIntkVlvActtionSystemOilPress\nj1939"]}, {"XNET Frame"="EFL_P4\nj1939", "Signals"=["EngAftercoolerCoolantLevel\nj1939", "EngCentrifugalOilFilterSpeed\nj1939", "EngChargeAirCooler1InletPress\nj1939", "EngChargeAirCooler2InletPress\nj1939", "EngChargeAirCoolerOutletPress\nj1939", "EngCoolantPumpDiffPress\nj1939", "EngIntercoolerCoolantLevel\nj1939"]}, {"XNET Frame"="EFL_P5\nj1939", "Signals"=["EngIntkVlvActtonOilPressForCyl1\nj1939", "EngIntkVlvActtonOilPressForCyl2\nj1939", "EngIntkVlvActtonOilPressForCyl3\nj1939", "EngIntkVlvActtonOilPressForCyl4\nj1939"]}, {"XNET Frame"="EFL_P6\nj1939", "Signals"=["EngIntkVlvActtonOilPressForCyl5\nj1939", "EngIntkVlvActtonOilPressForCyl6\nj1939", "EngIntkVlvActtonOilPressForCyl7\nj1939", "EngIntkVlvActtonOilPressForCyl8\nj1939"]}, {"XNET Frame"="EFL_P7\nj1939", "Signals"=["EngIntkVlvActtnOilPressForCyl10\nj1939", "EngIntkVlvActtnOilPressForCyl11\nj1939", "EngIntkVlvActtnOilPressForCyl12\nj1939", "EngIntkVlvActtonOilPressForCyl9\nj1939"]}, {"XNET Frame"="EFL_P8\nj1939", "Signals"=["EngIntkVlvActtnOilPressForCyl13\nj1939", "EngIntkVlvActtnOilPressForCyl14\nj1939", "EngIntkVlvActtnOilPressForCyl15\nj1939", "EngIntkVlvActtnOilPressForCyl16\nj1939"]}, {"XNET Frame"="EFL_P9\nj1939", "Signals"=["EngIntkVlvActtnOilPressForCyl17\nj1939", "EngIntkVlvActtnOilPressForCyl18\nj1939", "EngIntkVlvActtnOilPressForCyl19\nj1939", "EngIntkVlvActtnOilPressForCyl20\nj1939"]}, {"XNET Frame"="EFS\nj1939", "Signals"=["EngCoolantPreheatedState\nj1939", "EngFuelFilterSucSideDiffPress\nj1939", "EngFuelSupplyPumpInletPress\nj1939", "EngOilFilterOutletPress\nj1939", "EngOilLevelRemoteReservoir\nj1939", "EngOilPreHeatedState\nj1939", "EngOilPrimingPumpSwitch\nj1939", "EngOilPrimingState\nj1939", "EngVentilationStatus\nj1939", "EngWasteOilReservoirLevel\nj1939"]}, {"XNET Frame"="EGF1\nj1939", "Signals"=["EngExhstGsRcrcltionMassFlowRate\nj1939", "EngInletAirMassFlowRate\nj1939"]}, {"XNET Frame"="EGRBV\nj1939", "Signals"=["EGRCoolerBypassActuatorPostion\nj1939"]}, {"XNET Frame"="EH\nj1939", "Signals"=["TotalECUDistance\nj1939", "TotalECURunTime\nj1939"]}, {"XNET Frame"="EI\nj1939", "Signals"=["EngExhaustGasPress\nj1939", "EngFuelRackPos\nj1939", "EngMassFlow\nj1939", "EngPrefilterOilPress\nj1939", "InstantaneousEstBrakePower\nj1939"]}, {"XNET Frame"="EJM1\nj1939", "Signals"=["Joystick1GripXAxisPos\nj1939", "Joystick1GripYAxisPos\nj1939", "Joystick1ThetaAxisPos\nj1939", "Jystck1GripXAxisDetentPosStatus\nj1939", "Jystck1GripYAxisDetentPosStatus\nj1939", "Jystck1GrpXAxisNeutralPosStatus\nj1939", "Jystck1GrpXAxsLvrLftNgtvPsSttus\nj1939", "Jystck1GrpXAxsLvrRghtPstvPsStts\nj1939", "Jystck1GrpYAxisNeutralPosStatus\nj1939", "Jystck1GrpYAxsLvrBckNgtvPsSttus\nj1939", "Jystck1GrpYAxsLvrFrwrdPstvPsStts\nj1939", "Jystck1ThetaAxisDetentPosStatus\nj1939", "Jystck1ThtAxsClckwsPstvPsStatus\nj1939", "Jystck1ThtAxsCntrClckwsNgtvPsStt\nj1939", "Jystck1ThtaAxisNeutralPosStatus\nj1939"]}, {"XNET Frame"="EJM2\nj1939", "Signals"=["Joystick2GripXAxisPos\nj1939", "Joystick2GripYAxisPos\nj1939", "Joystick2ThetaAxisPos\nj1939", "Jystck2GripXAxisDetentPosStatus\nj1939", "Jystck2GripYAxisDetentPosStatus\nj1939", "Jystck2GrpXAxisNeutralPosStatus\nj1939", "Jystck2GrpXAxsLvrLftNgtvPsSttus\nj1939", "Jystck2GrpXAxsLvrRghtPstvPsStts\nj1939", "Jystck2GrpYAxisNeutralPosStatus\nj1939", "Jystck2GrpYAxsLvrBckNgtvPsSttus\nj1939", "Jystck2GrpYAxsLvrFrwrdPstvPsStts\nj1939", "Jystck2ThetaAxisDetentPosStatus\nj1939", "Jystck2ThtAxsClckwsPstvPsStatus\nj1939", "Jystck2ThtAxsCntrClckwsNgtvPsStt\nj1939", "Jystck2ThtaAxisNeutralPosStatus\nj1939"]}, {"XNET Frame"="EJM3\nj1939", "Signals"=["Joystick3GripXAxisPos\nj1939", "Joystick3GripYAxisPos\nj1939", "Joystick3ThetaAxisPos\nj1939", "Jystck3GripXAxisDetentPosStatus\nj1939", "Jystck3GripYAxisDetentPosStatus\nj1939", "Jystck3GrpXAxisNeutralPosStatus\nj1939", "Jystck3GrpXAxsLvrLftNgtvPsSttus\nj1939", "Jystck3GrpXAxsLvrRghtPstvPsStts\nj1939", "Jystck3GrpYAxisNeutralPosStatus\nj1939", "Jystck3GrpYAxsLvrBckNgtvPsSttus\nj1939", "Jystck3GrpYAxsLvrFrwrdPstvPsStts\nj1939", "Jystck3ThetaAxisDetentPosStatus\nj1939", "Jystck3ThtAxsClckwsPstvPsStatus\nj1939", "Jystck3ThtAxsCntrClckwsNgtvPsStt\nj1939", "Jystck3ThtaAxisNeutralPosStatus\nj1939"]}, {"XNET Frame"="EO1\nj1939", "Signals"=["EngActualExhaustOxygen\nj1939", "EngDesiredExhaustOxygen\nj1939", "EngDesiredRatedExhaustOxygen\nj1939", "EngExhstGsOxygnSnsrClsdLpOprton\nj1939", "EngExhstGsOxygnSnsrFlngCrrction\nj1939"]}, {"XNET Frame"="EOAC\nj1939", "Signals"=["TravelVelocityCtrlPos\nj1939"]}, {"XNET Frame"="EP\nj1939", "Signals"=["DataMemoryUsage\nj1939", "KeepAliveBatteryConsumption\nj1939"]}, {"XNET Frame"="EPD\nj1939", "Signals"=["PayloadPercentage\nj1939"]}, {"XNET Frame"="EPT1\nj1939", "Signals"=["EngExhaustGasPort1Temp\nj1939", "EngExhaustGasPort2Temp\nj1939", "EngExhaustGasPort3Temp\nj1939", "EngExhaustGasPort4Temp\nj1939"]}, {"XNET Frame"="EPT2\nj1939", "Signals"=["EngExhaustGasPort5Temp\nj1939", "EngExhaustGasPort6Temp\nj1939", "EngExhaustGasPort7Temp\nj1939", "EngExhaustGasPort8Temp\nj1939"]}, {"XNET Frame"="EPT3\nj1939", "Signals"=["EngExhaustGasPort10Temp\nj1939", "EngExhaustGasPort11Temp\nj1939", "EngExhaustGasPort12Temp\nj1939", "EngExhaustGasPort9Temp\nj1939"]}, {"XNET Frame"="EPT4\nj1939", "Signals"=["EngExhaustGasPort13Temp\nj1939", "EngExhaustGasPort14Temp\nj1939", "EngExhaustGasPort15Temp\nj1939", "EngExhaustGasPort16Temp\nj1939"]}, {"XNET Frame"="EPT5\nj1939", "Signals"=["EngExhaustGasPort17Temp\nj1939", "EngExhaustGasPort18Temp\nj1939", "EngExhaustGasPort19Temp\nj1939", "EngExhaustGasPort20Temp\nj1939"]}, {"XNET Frame"="ERC1\nj1939", "Signals"=["ActlMxAvlblRtarderPercentTorque\nj1939", "ActualRetarderPercentTorque\nj1939", "DrvrsDmandRetarderPercentTorque\nj1939", "EngCoolantLoadIncrease\nj1939", "IntendedRetarderPercentTorque\nj1939", "RetarderEnableBrakeAssistSwitch\nj1939", "RetarderEnableShiftAssistSwitch\nj1939", "RetarderRqingBrakeLight\nj1939", "RetarderSelectionNonEng\nj1939", "RetarderTorqueMode\nj1939", "SrcAddrssOfCtrllngDvcFrRtrdrCtrl\nj1939"]}, {"XNET Frame"="ERC2\nj1939", "Signals"=["TransOutputRetarder\nj1939"]}, {"XNET Frame"="ESC1\nj1939", "Signals"=["ActualInnerWheelSteerAngle\nj1939", "ESC1.AxleLocation\nj1939", "StatusOfSteerAxle\nj1939", "SteerType\nj1939", "SterableLiftAxleLoweringInhibit\nj1939", "TypeOfSteerForces\nj1939", "TypeOfSteerTrans\nj1939"]}, {"XNET Frame"="ESV1\nj1939", "Signals"=["EngSparkPlug1\nj1939", "EngSparkPlug2\nj1939", "EngSparkPlug3\nj1939", "EngSparkPlug4\nj1939"]}, {"XNET Frame"="ESV2\nj1939", "Signals"=["EngSparkPlug5\nj1939", "EngSparkPlug6\nj1939", "EngSparkPlug7\nj1939", "EngSparkPlug8\nj1939"]}, {"XNET Frame"="ESV3\nj1939", "Signals"=["EngSparkPlug10\nj1939", "EngSparkPlug11\nj1939", "EngSparkPlug12\nj1939", "EngSparkPlug9\nj1939"]}, {"XNET Frame"="ESV4\nj1939", "Signals"=["EngSparkPlug13\nj1939", "EngSparkPlug14\nj1939", "EngSparkPlug15\nj1939", "EngSparkPlug16\nj1939"]}, {"XNET Frame"="ESV5\nj1939", "Signals"=["EngSparkPlug17\nj1939", "EngSparkPlug18\nj1939", "EngSparkPlug19\nj1939", "EngSparkPlug20\nj1939"]}, {"XNET Frame"="ESV6\nj1939", "Signals"=["EngSparkPlug21\nj1939", "EngSparkPlug22\nj1939", "EngSparkPlug23\nj1939", "EngSparkPlug24\nj1939"]}, {"XNET Frame"="ET\nj1939", "Signals"=["EngExhstExhstGsTempLeftManifold\nj1939", "EngExhstExhstGsTmpRightManifold\nj1939"]}, {"XNET Frame"="ET1\nj1939", "Signals"=["EngCoolantTemp\nj1939", "EngFuelTemp\nj1939", "EngIntercoolerTemp\nj1939", "EngIntercoolerThermostatOpening\nj1939", "EngOilTemp1\nj1939", "EngTurboOilTemp\nj1939"]}, {"XNET Frame"="ET2\nj1939", "Signals"=["EngECUTemp\nj1939", "EngExhaustGasRecirculationTemp\nj1939", "EngExhstGsRcirculationDiffPress\nj1939", "EngOilTemp2\nj1939"]}, {"XNET Frame"="ET3\nj1939", "Signals"=["EngChargeAirCoolerOutletTemp\nj1939", "EngCoolantTempHiRes\nj1939", "EngIntakeManifold1AirTemp\nj1939", "EngIntkVlvActationSystemOilTemp\nj1939"]}, {"XNET Frame"="ETC1\nj1939", "Signals"=["EngMomentaryOverspeedEnable\nj1939", "ETC1.PercentClutchSlip\nj1939", "ProgressiveShiftDisable\nj1939", "SrcAddrssOfCtrllngDvcFrTrnsCtrl\nj1939", "TorqueConverterLockupEngaged\nj1939", "TransDrivelineEngaged\nj1939", "TransInputShaftSpeed\nj1939", "TransOutputShaftSpeed\nj1939", "TransShiftInProcess\nj1939"]}, {"XNET Frame"="ETC2\nj1939", "Signals"=["TransActualGearRatio\nj1939", "TransCurrentGear\nj1939", "TransCurrentRange\nj1939", "TransRqedRange\nj1939", "TransSelectedGear\nj1939"]}, {"XNET Frame"="ETC3\nj1939", "Signals"=["TransClutchActuator\nj1939", "TransDefuelActuator\nj1939", "TransInertiaBrakeActuator\nj1939", "TransLockupClutchActuator\nj1939", "TransRangeHighActuator\nj1939", "TransRangeLowActuator\nj1939", "TransShiftFingerGearActuator1\nj1939", "TransShiftFingerGearActuator2\nj1939", "TransShiftFingerGearPos\nj1939", "TransShiftFingerRailActuator1\nj1939", "TransShiftFingerRailActuator2\nj1939", "TransShiftFingerRailPos\nj1939", "TransSplitterDirectActuator\nj1939", "TransSplitterIndirectActuator\nj1939", "TrnsShftFngrCenterRailIndicator\nj1939", "TrnsShftFngrEngagementIndicator\nj1939", "TrnsShiftFingerNeutralIndicator\nj1939"]}, {"XNET Frame"="ETC4\nj1939", "Signals"=["TransSynchronizerBrakeValue\nj1939", "TransSynchronizerClutchValue\nj1939"]}, {"XNET Frame"="ETC5\nj1939", "Signals"=["TransForwardDirectionSwitch\nj1939", "TransHighRangeSenseSwitch\nj1939", "TransLowRangeSenseSwitch\nj1939", "TransNeutralSwitch\nj1939", "TransReverseDirectionSwitch\nj1939"]}, {"XNET Frame"="ETC6\nj1939", "Signals"=["ClutchLifeRemaining\nj1939", "HighestPossibleGear\nj1939", "LowestPossibleGear\nj1939", "RecommendedGear\nj1939"]}, {"XNET Frame"="ETC7\nj1939", "Signals"=["ActiveShiftConsoleIndicator\nj1939", "TransEngCrankEnable\nj1939", "TransMode1Indicator\nj1939", "TransMode2Indicator\nj1939", "TransMode3Indicator\nj1939", "TransMode4Indicator\nj1939", "TransReadyForBrakeRelease\nj1939", "TransRqedGearFeedback\nj1939", "TransRqedRangeDisplayBlankState\nj1939", "TransRqedRangeDisplayFlashState\nj1939", "TransShiftInhibitIndicator\nj1939"]}, {"XNET Frame"="ETC8\nj1939", "Signals"=["TransTorqueConverterRatio\nj1939"]}, {"XNET Frame"="FD\nj1939", "Signals"=["EstPercentFanSpeed\nj1939", "FanDriveState\nj1939", "FanSpeed\nj1939"]}, {"XNET Frame"="FL\nj1939", "Signals"=["EngFuelLeakage1\nj1939", "EngFuelLeakage2\nj1939"]}, {"XNET Frame"="FLI1\nj1939", "Signals"=["LaneDepartureImminentLeftSide\nj1939", "LaneDepartureImminentRightSide\nj1939"]}, {"XNET Frame"="FLI2\nj1939", "Signals"=["LaneTrackingStatusLeftSide\nj1939", "LaneTrackingStatusRightSide\nj1939", "LnDprtureIndicationEnableStatus\nj1939"]}, {"XNET Frame"="FLIC\nj1939", "Signals"=["LaneDepartureWarningEnableCmd\nj1939"]}, {"XNET Frame"="FMS\nj1939", "Signals"=["FMSstandardDiagnosticsSupported\nj1939", "FMSstandardRqsSupported\nj1939", "FMSstandardSWversionSupported\nj1939"]}, {"XNET Frame"="FWD\nj1939", "Signals"=["FrontWheelDriveActuatorStatus\nj1939"]}, {"XNET Frame"="FWSS1\nj1939", "Signals"=["FifthWheelDrawbarForce\nj1939", "FifthWheelRollMoment\nj1939", "FifthWheelRollWarningIndicator\nj1939", "FifthWheelVerticalForce\nj1939"]}, {"XNET Frame"="FWSS2\nj1939", "Signals"=["FfthWhlLckCoupleStatusIndicator\nj1939", "FfthWhlLckRadyToCoupleIndicator\nj1939", "FifthWheelErrorStatus\nj1939", "FifthWheelSliderLockIndicator\nj1939", "FifthWheelSliderPos\nj1939"]}, {"XNET Frame"="GAAC\nj1939", "Signals"=["GeneratorAverageACFrequency\nj1939", "GeneratorAverageACRMSCurrent\nj1939", "GnrtrAvrageLineLineACRMSVoltage\nj1939", "GnrtrAvrgLneNeutralACRMSVoltage\nj1939"]}, {"XNET Frame"="GFC\nj1939", "Signals"=["TotalFuelUsed\nj1939", "TripFuel\nj1939"]}, {"XNET Frame"="GFD\nj1939", "Signals"=["SpecificHeatRatio\nj1939"]}, {"XNET Frame"="GFI1\nj1939", "Signals"=["EngFuelSpecificGravity\nj1939", "GFI1.TotalEngPTOFuelUsed\nj1939", "GFI1.TripAverageFuelRate\nj1939"]}, {"XNET Frame"="GFI2\nj1939", "Signals"=["EngFuelFlowRate1\nj1939", "EngFuelFlowRate2\nj1939", "EngFuelValve1Pos\nj1939", "EngFuelValve2Pos\nj1939", "EngRqedFuelValve1Pos\nj1939", "EngRqedFuelValve2Pos\nj1939"]}, {"XNET Frame"="GFI3\nj1939", "Signals"=["EngFuelTemp2\nj1939", "EngFuelValve2InletAbsPress\nj1939", "EngFuelValve2OutletAbsPress\nj1939", "EngGasMassFlowRate2\nj1939"]}, {"XNET Frame"="GFP\nj1939", "Signals"=["EngAirToFuelDiffPress\nj1939", "EngFuelValve1OutletAbsPress\nj1939", "EngFuelValveDiffPress\nj1939", "EngFuelValveInletAbsPress\nj1939"]}, {"XNET Frame"="GPAAC\nj1939", "Signals"=["GeneratorPhaseAACFrequency\nj1939", "GeneratorPhaseAACRMSCurrent\nj1939", "GnrtrPhsALneNeutralACRMSVoltage\nj1939", "GnrtrPhseABLineLineACRMSVoltage\nj1939"]}, {"XNET Frame"="GPAACP\nj1939", "Signals"=["GeneratorPhaseAApparentPower\nj1939", "GeneratorPhaseARealPower\nj1939"]}, {"XNET Frame"="GPAACR\nj1939", "Signals"=["GeneratorPhaseAPowerFactor\nj1939", "GeneratorPhaseAReactivePower\nj1939", "GnratorPhaseAPowerFactorLagging\nj1939"]}, {"XNET Frame"="GPBAC\nj1939", "Signals"=["GeneratorPhaseBACFrequency\nj1939", "GeneratorPhaseBACRMSCurrent\nj1939", "GnrtrPhsBLneNeutralACRMSVoltage\nj1939", "GnrtrPhseBCLineLineACRMSVoltage\nj1939"]}, {"XNET Frame"="GPBACP\nj1939", "Signals"=["GeneratorPhaseBApparentPower\nj1939", "GeneratorPhaseBRealPower\nj1939"]}, {"XNET Frame"="GPBACRP\nj1939", "Signals"=["GeneratorPhaseBPowerFactor\nj1939", "GeneratorPhaseBReactivePower\nj1939", "GnratorPhaseBPowerFactorLagging\nj1939"]}, {"XNET Frame"="GPCAC\nj1939", "Signals"=["GeneratorPhaseCACFrequency\nj1939", "GeneratorPhaseCACRMSCurrent\nj1939", "GnrtrPhsCLneNeutralACRMSVoltage\nj1939", "GnrtrPhseCALineLineACRMSVoltage\nj1939"]}, {"XNET Frame"="GPCACP\nj1939", "Signals"=["GeneratorPhaseCApparentPower\nj1939", "GeneratorPhaseCRealPower\nj1939"]}, {"XNET Frame"="GPCACR\nj1939", "Signals"=["GeneratorPhaseCPowerFactor\nj1939", "GeneratorPhaseCReactivePower\nj1939", "GnratorPhaseCPowerFactorLagging\nj1939"]}, {"XNET Frame"="GPM11\nj1939", "Signals"=["AntiTheftDeviceReq\nj1939", "ODDRequest\nj1939", "GPM11.VehicleType\nj1939"]}, {"XNET Frame"="GPM12\nj1939", "Signals"=["EngineSpeedLowerLimit\nj1939", "EngineSpeedUpperLimit\nj1939", "GPM12.MaxVehicleSpeedLimit\nj1939"]}, {"XNET Frame"="GPM13\nj1939", "Signals"=["ActualEngine_PercTorque\nj1939", "DriversDemandEngine_PercTorque\nj1939", "EngineControlAllowed\nj1939", "EngineRunning\nj1939", "EngineSpeed\nj1939", "EngineTorqueMode\nj1939", "PercentLoadAtCurrentSpeed\nj1939", "VehicleSpeed\nj1939"]}, {"XNET Frame"="GPM14\nj1939", "Signals"=["AccelPedalLowIdleSwitch\nj1939", "AccelPedalPosition\nj1939", "ClutchIndptdPTOFeedback\nj1939", "CurrentGear\nj1939", "FirstClutchDpdtPTOFeedback\nj1939", "FirstEngineMtdPTOFeedback\nj1939", "PTOControlAllowed\nj1939", "GPM14.PercentClutchSlip\nj1939", "SecClutchDptdPTOFeedback\nj1939", "SecEngineMtdPTOFeedback\nj1939", "StarterActive\nj1939", "TorqueConvOilTemp\nj1939", "TorqueConvtOilTempWarning\nj1939"]}, {"XNET Frame"="GPM15\nj1939", "Signals"=["EngineCoolantTempWarning\nj1939", "GPM15.EngineCoolantTemperature\nj1939", "EngineOilPressure\nj1939", "EngineOilPressureWarning\nj1939", "EngineOilTemperature\nj1939", "FuelLevelWarning\nj1939", "ReferenceEngineTorque\nj1939"]}, {"XNET Frame"="GPM16\nj1939", "Signals"=["AmbientAirTemperature\nj1939"]}, {"XNET Frame"="GPM21\nj1939", "Signals"=["GPM21.VehicleType\nj1939"]}, {"XNET Frame"="GPM22\nj1939", "Signals"=["AntiTheftDeviceStatus\nj1939", "BodyFluidLevel\nj1939", "BodyPressure\nj1939", "ODDStatus\nj1939", "RearObstacleDistance\nj1939", "ThermalBodyTemperature\nj1939"]}, {"XNET Frame"="GPM23\nj1939", "Signals"=["ReqEngineSpeed\nj1939", "ReqEngineSpeedLimit\nj1939", "ReqEngineSpeedLowerLim\nj1939", "ReqEngineSpeedUpperLim\nj1939", "ReqEngineTorqueLimit\nj1939"]}, {"XNET Frame"="GPM24\nj1939", "Signals"=["ClutchIndpdtPTOSwitch\nj1939", "EngineStartSwitch\nj1939", "EngineStopSwitch\nj1939", "FirstClutchDpdtPTOSwitch\nj1939", "FirstEngineMtdPTOSwitch\nj1939", "OperatingPanelActive\nj1939", "RefusePackerStepSwitch\nj1939", "RqstedPercentClutchSlip\nj1939", "SecClutchDpdtPTOSwitch\nj1939", "SecEngineMtdPTOSwitch\nj1939", "StarterLockoutSwitch\nj1939"]}, {"XNET Frame"="GPM25\nj1939", "Signals"=["TrailRightRearWidIndLight\nj1939", "TrailerInteriorLight\nj1939", "TrailerLeftCrnMarkerLight\nj1939", "TrailerLeftDirIndLight\nj1939", "TrailerLeftRearFogLight\nj1939", "TrailerLeftRearLight\nj1939", "TrailerLeftRearRegPltLight\nj1939", "TrailerLeftRearWidIndLight\nj1939", "TrailerLeftReversingLight\nj1939", "TrailerLeftSideMarkerLight\nj1939", "TrailerLeftStopLight\nj1939", "TrailerRearWarningLight\nj1939", "TrailerRightCrnMarkerLight\nj1939", "TrailerRightDirIndLight\nj1939", "TrailerRightRearFogLight\nj1939", "TrailerRightRearLight\nj1939", "TrailerRightRearRegPltLight\nj1939", "TrailerRightReversingLight\nj1939", "TrailerRightSideMrkLight\nj1939", "TrailerRightStopLight\nj1939", "TrailerRotatingIdentLight\nj1939", "TrailerWorkLamp\nj1939"]}, {"XNET Frame"="GTACE\nj1939", "Signals"=["GeneratorTotalKWHoursExport\nj1939", "GeneratorTotalKWHoursImport\nj1939"]}, {"XNET Frame"="GTACP\nj1939", "Signals"=["GeneratorTotalApparentPower\nj1939", "GeneratorTotalRealPower\nj1939"]}, {"XNET Frame"="GTACR\nj1939", "Signals"=["GeneratorOverallPowerFactor\nj1939", "GeneratorTotalReactivePower\nj1939", "GnrtorOverallPowerFactorLagging\nj1939"]}, {"XNET Frame"="HBS\nj1939", "Signals"=["HydBrakeFluidLevelSwitch\nj1939", "HydBrakePressCircuit1\nj1939", "HydBrakePressCircuit2\nj1939", "HydBrakeSystemAudibleWarningCmd\nj1939", "HydBrkPressWarningStateCircuit1\nj1939", "HydBrkPressWarningStateCircuit2\nj1939", "HydBrkePressSupplyStateCircuit1\nj1939", "HydBrkePressSupplyStateCircuit2\nj1939"]}, {"XNET Frame"="HOURS\nj1939", "Signals"=["EngTotalHoursOfOperation\nj1939", "EngTotalRevolutions\nj1939"]}, {"XNET Frame"="HPG\nj1939", "Signals"=["EngHydPressGovernorSwitch\nj1939", "EngHydPrssGovernorModeIndicator\nj1939", "FireApparatusPumpEngagement\nj1939", "HydPress\nj1939"]}, {"XNET Frame"="HRW\nj1939", "Signals"=["FrontAxleLeftWheelSpeed\nj1939", "FrontAxleRightWheelSpeed\nj1939", "RearAxleLeftWheelSpeed\nj1939", "RearAxleRightWheelSpeed\nj1939"]}, {"XNET Frame"="HTR\nj1939", "Signals"=["AuxHeaterInputAirTemp\nj1939", "AuxHeaterMode\nj1939", "AuxHeaterOutputCoolantTemp\nj1939", "AuxHeaterOutputPowerPercent\nj1939", "AuxilaryHeaterWaterPumpStatus\nj1939", "CabHeatingZone\nj1939", "CabVentilation\nj1939", "EngHeatingZone\nj1939"]}, {"XNET Frame"="IC1\nj1939", "Signals"=["EngAirFilter1DiffPress\nj1939", "EngAirInletPress\nj1939", "EngCoolantFilterDiffPress\nj1939", "EngExhaustGasTemp\nj1939", "EngIntakeManifold1Temp\nj1939", "EngParticulateTrapInletPress\nj1939", "IC1.EngTurboBoostPress\nj1939"]}, {"XNET Frame"="IC2\nj1939", "Signals"=["EngAirFilter2DiffPress\nj1939", "EngAirFilter3DiffPress\nj1939", "EngAirFilter4DiffPress\nj1939", "EngIntakeManifold1AbsPress\nj1939", "EngIntakeManifold2Press\nj1939"]}, {"XNET Frame"="IMT1\nj1939", "Signals"=["EngTurbo1BoostPress\nj1939", "EngTurbo2BoostPress\nj1939", "EngTurbo3BoostPress\nj1939", "EngTurbo4BoostPress\nj1939"]}, {"XNET Frame"="IMT2\nj1939", "Signals"=["EngIntakeManifold2Temp\nj1939", "EngIntakeManifold3Temp\nj1939", "EngIntakeManifold4Temp\nj1939", "EngIntakeManifold5Temp\nj1939", "EngIntakeManifold6Temp\nj1939"]}, {"XNET Frame"="IO\nj1939", "Signals"=["EngTotalIdleFuelUsed\nj1939", "EngTotalIdleHours\nj1939"]}, {"XNET Frame"="ISC\nj1939", "Signals"=["EngOprtrPrmryIntrmdtSpeedSelect\nj1939"]}, {"XNET Frame"="ISCS\nj1939", "Signals"=["EngOprtrPrmryIntrmdtSpdSlctStte\nj1939"]}, {"XNET Frame"="ISO1\nj1939", "Signals"=["EngCyl1IgntTransSecondOutput\nj1939", "EngCyl2IgntTransSecondOutput\nj1939", "EngCyl3IgntTransSecondOutput\nj1939", "EngCyl4IgntTransSecondOutput\nj1939", "EngCyl5IgntTransSecondOutput\nj1939", "EngCyl6IgntTransSecondOutput\nj1939", "EngCyl7IgntTransSecondOutput\nj1939", "EngCyl8IgntTransSecondOutput\nj1939"]}, {"XNET Frame"="ISO15765_Funct\nj1939", "Signals"=["ISO15765_Funct.BlockSize\nj1939", "ISO15765_Funct.FirstFrameDataLength\nj1939", "ISO15765_Funct.FlowStatus\nj1939", "ISO15765_Funct.ProtocolCtrlInformation\nj1939", "ISO15765_Funct.SN\nj1939", "ISO15765_Funct.SeparationTime\nj1939", "ISO15765_Funct.SingleFrameDataLength\nj1939"]}, {"XNET Frame"="ISO15765_Phys\nj1939", "Signals"=["ISO15765_Phys.BlockSize\nj1939", "ISO15765_Phys.FirstFrameDataLength\nj1939", "ISO15765_Phys.FlowStatus\nj1939", "ISO15765_Phys.ProtocolCtrlInformation\nj1939", "ISO15765_Phys.SN\nj1939", "ISO15765_Phys.SeparationTime\nj1939", "ISO15765_Phys.SingleFrameDataLength\nj1939"]}, {"XNET Frame"="ISO2\nj1939", "Signals"=["EngCyl10IgntTransSecondOutput\nj1939", "EngCyl11IgntTransSecondOutput\nj1939", "EngCyl12IgntTransSecondOutput\nj1939", "EngCyl13IgntTransSecondOutput\nj1939", "EngCyl14IgntTransSecondOutput\nj1939", "EngCyl15IgntTransSecondOutput\nj1939", "EngCyl16IgntTransSecondOutput\nj1939", "EngCyl9IgntTransSecondOutput\nj1939"]}, {"XNET Frame"="ISO3\nj1939", "Signals"=["EngCyl17IgntTransSecondOutput\nj1939", "EngCyl18IgntTransSecondOutput\nj1939", "EngCyl19IgntTransSecondOutput\nj1939", "EngCyl20IgntTransSecondOutput\nj1939"]}, {"XNET Frame"="IT1\nj1939", "Signals"=["EngCyl1IgntTiming\nj1939", "EngCyl2IgntTiming\nj1939", "EngCyl3IgntTiming\nj1939", "EngCyl4IgntTiming\nj1939"]}, {"XNET Frame"="IT2\nj1939", "Signals"=["EngCyl5IgntTiming\nj1939", "EngCyl6IgntTiming\nj1939", "EngCyl7IgntTiming\nj1939", "EngCyl8IgntTiming\nj1939"]}, {"XNET Frame"="IT3\nj1939", "Signals"=["EngCyl10IgntTiming\nj1939", "EngCyl11IgntTiming\nj1939", "EngCyl12IgntTiming\nj1939", "EngCyl9IgntTiming\nj1939"]}, {"XNET Frame"="IT4\nj1939", "Signals"=["EngCyl13IgntTiming\nj1939", "EngCyl14IgntTiming\nj1939", "EngCyl15IgntTiming\nj1939", "EngCyl16IgntTiming\nj1939"]}, {"XNET Frame"="IT5\nj1939", "Signals"=["EngCyl17IgntTiming\nj1939", "EngCyl18IgntTiming\nj1939", "EngCyl19IgntTiming\nj1939", "EngCyl20IgntTiming\nj1939"]}, {"XNET Frame"="IT6\nj1939", "Signals"=["EngActualIgntTiming\nj1939", "EngDesiredIgntTiming1\nj1939", "EngDesiredIgntTiming2\nj1939", "EngDesiredIgntTiming3\nj1939"]}, {"XNET Frame"="J2012\nj1939", "Signals"=["J2012DTCOccurrenceCount\nj1939", "J2012DTCStatus\nj1939", "NumberOfJ2012DTCs\nj1939"]}, {"XNET Frame"="KL1\nj1939", "Signals"=["EngCyl1KnockLevel\nj1939", "EngCyl2KnockLevel\nj1939", "EngCyl3KnockLevel\nj1939", "EngCyl4KnockLevel\nj1939", "EngCyl5KnockLevel\nj1939", "EngCyl6KnockLevel\nj1939", "EngCyl7KnockLevel\nj1939", "EngCyl8KnockLevel\nj1939"]}, {"XNET Frame"="KL2\nj1939", "Signals"=["EngCyl10KnockLevel\nj1939", "EngCyl11KnockLevel\nj1939", "EngCyl12KnockLevel\nj1939", "EngCyl13KnockLevel\nj1939", "EngCyl14KnockLevel\nj1939", "EngCyl15KnockLevel\nj1939", "EngCyl16KnockLevel\nj1939", "EngCyl9KnockLevel\nj1939"]}, {"XNET Frame"="KL3\nj1939", "Signals"=["EngCyl17KnockLevel\nj1939", "EngCyl18KnockLevel\nj1939", "EngCyl19KnockLevel\nj1939", "EngCyl20KnockLevel\nj1939", "EngCyl21KnockLevel\nj1939", "EngCyl22KnockLevel\nj1939", "EngCyl23KnockLevel\nj1939", "EngCyl24KnockLevel\nj1939"]}, {"XNET Frame"="LBC\nj1939", "Signals"=["BladeCtrlMode\nj1939", "BladeDurationAndDirection\nj1939"]}, {"XNET Frame"="LC\nj1939", "Signals"=["AltBeamHeadLightCmd\nj1939", "BackUpLightAndAlarmHornCmd\nj1939", "CenterStopLightCmd\nj1939", "HighBeamHeadLightCmd\nj1939", "ImplementClearanceLightCmd\nj1939", "ImplementLeftFacingWorkLightCmd\nj1939", "ImplementMarkerLightCmd\nj1939", "ImplementOEMOption1LightCmd\nj1939", "ImplementOEMOption2LightCmd\nj1939", "ImplementRearWorkLightCmd\nj1939", "ImplmentLeftForwardWorkLightCmd\nj1939", "ImplmentRightFacingWorkLightCmd\nj1939", "ImplmntRightForwardWorkLightCmd\nj1939", "LeftStopLightCmd\nj1939", "LeftTurnSignalLightsCmd\nj1939", "LightingDataRqCmd\nj1939", "LowBeamHeadLightCmd\nj1939", "RearFogLightCmd\nj1939", "RightStopLightCmd\nj1939", "RightTurnSignalLightsCmd\nj1939", "RotatingBeaconLightCmd\nj1939", "RunningLightCmd\nj1939", "TractorClearanceLightCmd\nj1939", "TractorFrontFogLightsCmd\nj1939", "TractorMarkerLightCmd\nj1939", "TrctrFrntHghMuntedWorkLightsCmd\nj1939", "TrctrFrntLwMountedWorkLightsCmd\nj1939", "TrctrRarLowMountedWorkLightsCmd\nj1939", "TrctrRrHighMountedWorkLightsCmd\nj1939", "TrctrSdHighMountedWorkLightsCmd\nj1939", "TrctrSdeLowMountedWorkLightsCmd\nj1939", "TrctrUndrsdMountedWorkLightsCmd\nj1939"]}, {"XNET Frame"="LD\nj1939", "Signals"=["AltBeamHeadLightData\nj1939", "BackUpLightAndAlarmHorn\nj1939", "CenterStopLight\nj1939", "HighBeamHeadLightData\nj1939", "ImplementClearanceLight\nj1939", "ImplementLeftFacingWorkLight\nj1939", "ImplementLeftForwardWorkLight\nj1939", "ImplementMarkerLight\nj1939", "ImplementOEMOption1Light\nj1939", "ImplementOEMOption2Light\nj1939", "ImplementRearWorkLight\nj1939", "ImplementRightFacingWorkLight\nj1939", "ImplementRightForwardWorkLight\nj1939", "LeftStopLight\nj1939", "LeftTurnSignalLights\nj1939", "LowBeamHeadLightData\nj1939", "RearFogLights\nj1939", "RightStopLight\nj1939", "RightTurnSignalLights\nj1939", "RotatingBeaconLight\nj1939", "RunningLight\nj1939", "TractorClearanceLight\nj1939", "TractorFrontFogLights\nj1939", "TractorMarkerLight\nj1939", "TractorRearLowMountedWorkLights\nj1939", "TractorSideLowMountedWorkLights\nj1939", "TrctorFrontLowMountedWorkLights\nj1939", "TrctorRearHighMountedWorkLights\nj1939", "TrctorSideHighMountedWorkLights\nj1939", "TrctrFrontHighMountedWorkLights\nj1939", "TrctrUndersideMountedWorkLights\nj1939"]}, {"XNET Frame"="LFC\nj1939", "Signals"=["EngTotalFuelUsed\nj1939", "EngTripFuel\nj1939"]}, {"XNET Frame"="LFE\nj1939", "Signals"=["EngAverageFuelEconomy\nj1939", "EngFuelRate\nj1939", "EngInstantaneousFuelEconomy\nj1939", "EngThrottle2Pos\nj1939", "EngThrottlePos\nj1939"]}, {"XNET Frame"="LFI\nj1939", "Signals"=["LFI.TotalEngPTOFuelUsed\nj1939", "LFI.TripAverageFuelRate\nj1939"]}]
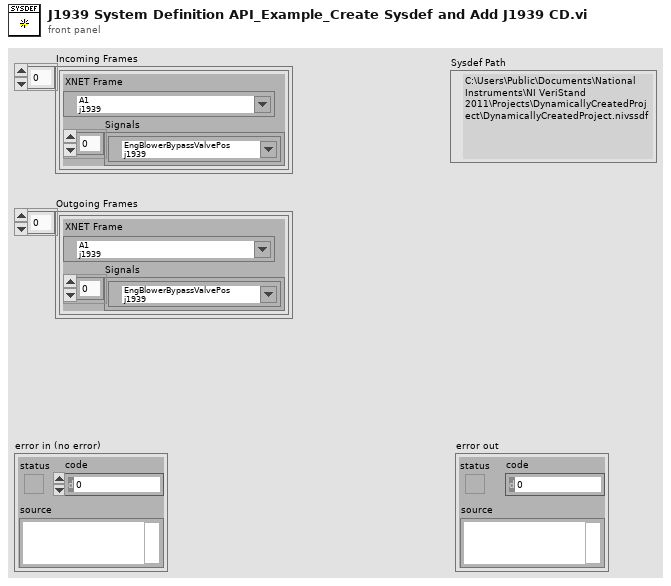
[diagram p1: front panel]
types:
  T1 = typedef "J1939 System Definition API.lvlibp/J1939 System Definition API Support.lvlib/Add Item - Frame Cluster.ctl" = cluster{"XNET Frame":refnum<k21>, "Signals":refnum<k21>[]}
  T2 = typedef "J1939 System Definition API.lvlibp/J1939 System Definition API Support.lvlib/Remove Frame Action.ctl" = enum16{"Incoming", "Outgoing"}
  T3 = typedef "J1939 System Definition API.lvlibp/J1939 Addon Shared.lvlib/Monitor Settings.ctl" = cluster{"J1939 Network Address":u8, "Name":u64}
  T4 = typedef "J1939 System Definition API.lvlibp/J1939 Addon Shared.lvlib/XNET Settings.ctl" = cluster{"XNET Database":refnum<k21>, "XNET Cluster":refnum<k21>, "CAN Port":string, "Baud rate [Bd]":u32, "Termination":u32, "Incoming Rate":u32, "Outcoming Rate":u32, "Write Decimation":u32}
  T5 = typedef "J1939 System Definition API.lvlibp/Custom Device API.lvlib/Custom Device Item Ref.ctl" = u64
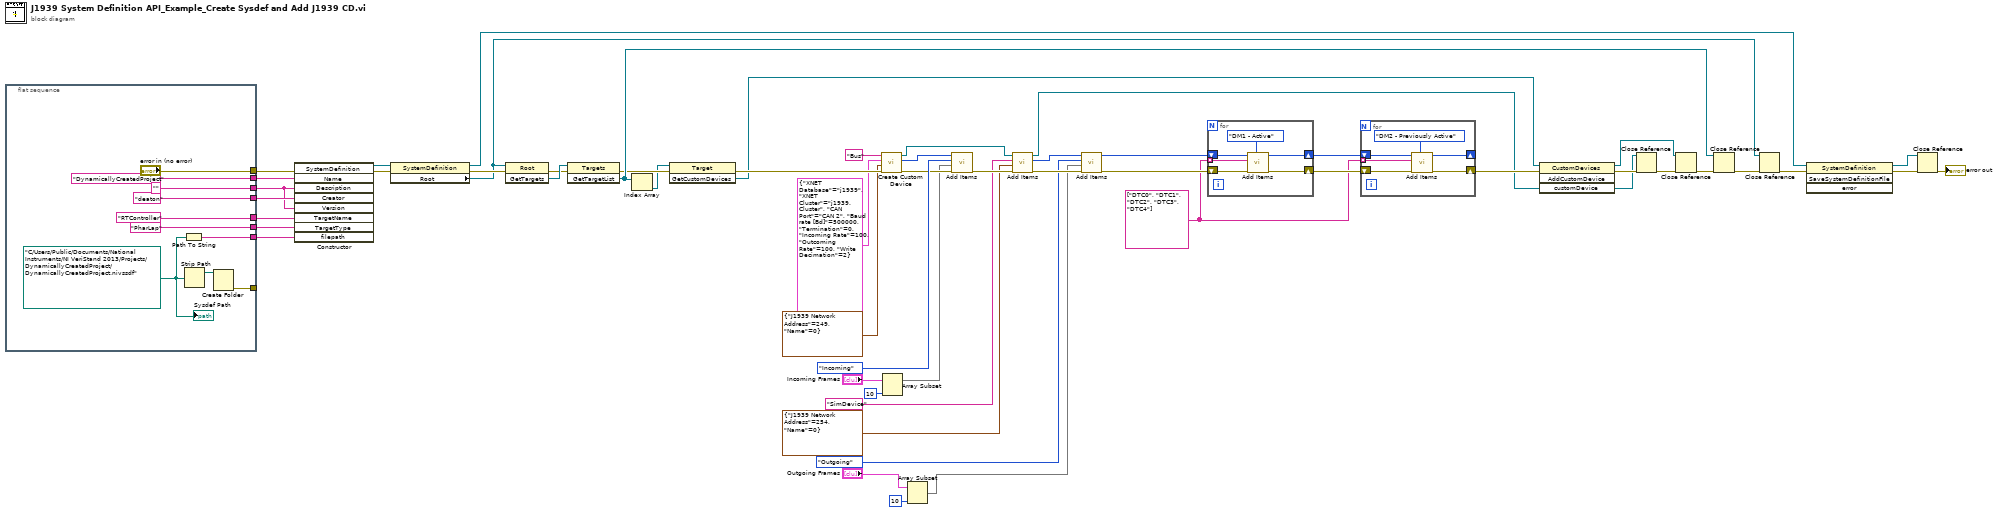
[diagram p0: block diagram]
diagram:
  w7 = string[] ["DTC0", "DTC1", "DTC2", "DTC3", "DTC4"]
  n1 = flat-sequence {
    tunnel: ["DynamicallyCreatedProject" ("Name")] -> w54
    tunnel: ["deaton" ("Creator")] -> w53
    tunnel: ["RTController" ("TargetName")] -> w38
    tunnel: ["PharLap" ("TargetType")] -> w52
    tunnel: ["" ("Description")] -> w51
    tunnel: [w57] -> w50
    tunnel: [w56] -> _
    tunnel: ["error in (no error)"] -> w39
    frame #0 {
      w58 = path "C:/Users/Public/Documents/National Instruments/NI VeriStand 2013/Projects/DynamicallyCreatedProject/DynamicallyCreatedProject.nivssdf"
      n2 = Path To String(path=w58) -> (string=w57:string)
      n3 = Strip Path(path=w58) -> (stripped path=w59:path)  [unwired: 1 out]
      n4 = Create Folder(path (use dialog)=w59) -> (error out=w56:errorcluster)  [unwired: 2 in, 2 out]
      "Sysdef Path" <- w58
    }
  }
  n5 = constructor class="SystemDefinition"(error in=w39, "Name"=w54, "Description"=w51, "Creator"=w53, "Version"=w51, "TargetName"=w38, "TargetType"=w52, "filepath"=w50) -> (reference out=w45:refnum<k24>, error out=w48:errorcluster)  [unwired: 2 in, 8 out]
  n6 = property class="SystemDefinition"(reference=w45, error in=w48) -> (reference out=w44:refnum<k24>, error out=w47:errorcluster, "Root"=w35:refnum<k24>)
  n7 = invoke class="Root" method="GetTargets"(reference=w35, error in=w47) -> (error out=w43:errorcluster, "GetTargets"=w49:refnum<k24>)  [unwired: 1 in, 1 out]
  n8 = invoke class="Targets" method="GetTargetList"(reference=w49, error in=w43) -> (error out=w31:errorcluster, "GetTargetList"=w46:refnum<k24>[])  [unwired: 1 in, 1 out]
  n9 = Index Array(array=w46) -> (element=w30:refnum<k24>)  [unwired: 1 in]
  n10 = invoke class="Target" method="GetCustomDevices"(reference=w30, error in=w31) -> (error out=w33:errorcluster, "GetCustomDevices"=w32:refnum<k24>)  [unwired: 1 in, 1 out]
  n11 = call "Create Custom Device.vi"("error in (no error)"=w33, "J1939 Monitor Settings"=T3 {"J1939 Network Address"=249, "Name"=0}, "J1939 XNET Settings"=T4 {"XNET Database"="j1939", "XNET Cluster"="j1939.Cluster", "CAN Port"="CAN 2", "Baud rate [Bd]"=500000, "Termination"=0, "Incoming Rate"=100, "Outcoming Rate"=100, "Write Decimation"=2}, "Name"="Bus") -> ("error out"=w26:errorcluster, "Monitor Ref out"=w24:T5, "Custom Device reference"=w16:refnum<k24>)  [unwired: 5 in]
  n12 = Array Subset(array="Incoming Frames", length=10) -> (w6:T1[])  [unwired: 1 in]
  n13 = Array Subset(array="Outgoing Frames", length=10) -> (w2:T1[])  [unwired: 1 in]
  n14 = call-poly "Add Items.vi"("error in (no error)"=w26, "Frames"=w6, "Action"=Remove_Frame_Action."Incoming", "Section Ref in"=w24) -> ("error out"=w22:errorcluster)  [unwired: 6 in, 1 out]
  n15 = call-poly "Add Items.vi"("error in (no error)"=w22, "J1939 Monitor Settings"=T3 {"J1939 Network Address"=254, "Name"=0}, "Name"="SimDevice", "Custom Device reference in"=w16) -> ("error out"=w19:errorcluster, "Device Ref out"=w17:T5, "Custom Device reference out"=w15:refnum<k24>)  [unwired: 5 in]
  n16 = call-poly "Add Items.vi"("error in (no error)"=w19, "Frames"=w2, "Action"=Remove_Frame_Action."Outgoing", "Section Ref in"=w17) -> ("error out"=w18:errorcluster, "Section Ref out"=w11:T5)  [unwired: 6 in]
  n17 = for {
    shift-right: [w70] -> w21
    shift-left: w18 -> [w69]
    shift-right: [w66] -> w14
    shift-left: w11 -> [w67]
    tunnel: w7 -> [w65] mode=indexing
    n18 = call-poly "Add Items.vi"("DTC Type"=enum8{"DM1 - Active", "DM2 - Previously Active"}."DM1 - Active", "error in (no error)"=w69, "Name"=w65, "Device Ref in"=w67) -> ("error out"=w70:errorcluster, "Device Ref out"=w66:T5)  [unwired: 6 in]
  }
  n19 = for {
    shift-right: [w75] -> w20
    shift-left: w21 -> [w76]
    shift-right: [w72] -> _
    shift-left: w14 -> [w73]
    tunnel: w7 -> [w71] mode=indexing
    n20 = call-poly "Add Items.vi"("DTC Type"=enum8{"DM1 - Active", "DM2 - Previously Active"}."DM2 - Previously Active", "error in (no error)"=w76, "Name"=w71, "Device Ref in"=w73) -> ("error out"=w75:errorcluster, "Device Ref out"=w72:T5)  [unwired: 6 in]
  }
  n21 = invoke class="CustomDevices" method="AddCustomDevice"(reference=w32, error in=w20, "customDevice"=w15) -> (reference out=w9:refnum<k24>, error out=w29:errorcluster)  [unwired: 1 in, 2 out]
  n22 = Close Reference(reference=w15, error in (no error)=w29) -> (error out=w8:errorcluster)
  n23 = Close Reference(reference=w9, error in (no error)=w8) -> (error out=w28:errorcluster)
  n24 = Close Reference(reference=w46, error in (no error)=w28) -> (error out=w36:errorcluster)
  n25 = Close Reference(reference=w35, error in (no error)=w36) -> (error out=w34:errorcluster)
  n26 = invoke class="SystemDefinition" method="SaveSystemDefinitionFile"(reference=w44, error in=w34) -> (reference out=w40:refnum<k24>, error out=w42:errorcluster)  [unwired: 2 in, 2 out]
  n27 = Close Reference(reference=w40, error in (no error)=w42) -> (error out=→"error out":errorcluster)
